vi "PECT - Scan_time gate_counter -XSeries-DAQ Pulser.vi"() -> ()   [LabVIEW 2018]
uses:
  <vilib>/DAQmx/read.llb/DAQmx Read (Counter U32 1Chan 1Samp).vi
  <vilib>/DAQmx/write.llb/DAQmx Write (Analog Wfm 1Chan NSamp).vi
  <vilib>/DAQmx/read.llb/DAQmx Read (Analog 1D DBL 1Chan NSamp).vi
  <vilib>/DAQmx/read.llb/DAQmx Read (Analog Wfm 1Chan NSamp).vi
  <vilib>/Instr/_visa.llb/VISA Configure Serial Port (Instr).vi
  <vilib>/DAQmx/create/channels.llb/DAQmx Create Channel (AI-Voltage-Basic).vi
  <vilib>/DAQmx/create/channels.llb/DAQmx Create Channel (CI-Count Edges).vi
  <vilib>/DAQmx/miscellaneous.llb/DAQmx Fill In Error Info.vi
  <vilib>/DAQmx/configure/timing.llb/DAQmx Timing (Sample Clock).vi
  <vilib>/DAQmx/configure/trigger.llb/DAQmx Start Trigger (Digital Edge).vi
  <vilib>/DAQmx/create/channels.llb/DAQmx Create Channel (AO-Voltage-Basic).vi
  Global_data.vi
  <vilib>/express/express analysis/Spectral/Block/exnSpectralBlock spectral measurements PSD poly.vi
  <vilib>/express/express analysis/Spectral/Block/exnSpectralBlock spectral measurements PSD WFM.vi
  <vilib>/express/express analysis/Spectral/XNode/ExpressSpectralMeasurementsBlockNode.xnode
  <resource>/objmgr/daqmx.rc
  <vilib>/measure/NI_MABase.lvlib
  <vilib>/Platform/NI_3dgraph.lvlib
  <vilib>/DAQmx/write.llb/DAQmx Write (Analog 1D Wfm NChan NSamp).vi
panel:
  in  "Tab Control 3":enum32{"Control", "Data Processing"}(tab)
  in  "Duty cycle %":dbl=50.0 format="%#.2f"
  in  "Pulser Trigger":tag="/Dev6/PFI0"
  in  "Edge":i32(ring)=10280 items=["Rising"=10280, "Falling"=10171]
  in  "2 Plots":bool
  in  "Offset":bool
  in  "Open csv":bool
  in  "Scan":bool
  in  "Save Scan mode":bool caption="Save Process"
  in  "Gate 1":dbl
  in  "Gate 2":dbl=50.0
  in  "Stop Scan":bool
  in  "Right":bool
  in  "Left":bool
  in  "Front":bool
  in  "Back":bool
  in  "Home X":bool
  in  "Home Y":bool
  in  "Stop 3":bool
  in  "Emergency Stop":bool
  in  "Move Distance":dbl=5.0
  in  "Pulse generator":T1={"Waveform Type"=2, "Amplitude"=10.0, "Frequency"=1000.0} {"Frequency" format="%0.2p"; "Amplitude" format="%0.2p"; "Waveform Type" items=["Sine Wave", "Triangle Wave", "Square Wave", "Sawtooth Wave"]}
  in  "Open tdms":bool
  in  "Motor Counter Terminal":tag="PFI8"
  in  "Motor counter":tag="Dev6/ctr0"
  out "Motor Pulse Count":i32
  in  "Cursor":bool=TRUE
  in  "Repair Line Col":bool
  in  "Repair Line Row":bool
  in  "Line Col":dbl=167.0
  in  "Line Row":dbl
  in  "Y-max":dbl
  in  "Y-min":dbl
  in  "X-max":dbl
  in  "X-min":dbl
  in  "Inverse":bool caption="Scan"
  in  "ViewMode":i32(ring) items=["cwViewXYPlane", "cwViewXZPlane", "cwViewYZPlane", "cwViewUserDefined"]
  in  "Plot style":i32(ring)=5 items=["cwLine"=1, "cwPoint"=2, "cwLinePoint"=3, "cwHiddenLine"=4, "cwSurface"=5, "cwSurfaceLine"=6, "cwSurfaceNormal"=7, "cwContourLine"=8, "cwSurfaceContour"=9]
  in  "ColorMapAutoScale":bool=TRUE
  in  "Max":dbl=0.6
  in  "Min":dbl=-0.8
  in  "low cutoff freq: fl":dbl=40.0 format="%0.2f"
  in  "Filter":bool caption="Scan"
  in  "Backindex":i32
  in  "Backdata":bool caption="Scan"
  in  "Odd":bool caption="Scan"
  in  "DiffX":bool caption="Scan"
  in  "DiffY":bool caption="Scan"
  in  "Abs":bool caption="Scan"
  in  "Trim data":bool caption="Scan"
  in  "Return":bool caption="Scan"
  out "Start Pos. X":dbl=-22.5 format="%#.4f"
  out "Start. Pos.Y":dbl=18.8 format="%#.4f"
  out "No.data":i32
  in  "Stop 4":bool
  in  "Tab Control 2":T2(tab)
  out "Hall sensors signal":waveform(dbl)[](graph)=[{"t0"=timestamp(3525645621.636764 s since 1904-01-01), "dt"=1.9999999999999944e-06, "Y"=array[2100 elements], "attributes"=variant("NI_ChannelName"=variant(string "Dev1/ai0"), "NI_UnitDescription"=variant(string "Volts"))}, {"t0"=timestamp(3525645621.636764 s since 1904-01-01), "dt"=1.9999999999999944e-06, "Y"=array[2100 elements], "attributes"=variant("NI_ChannelName"=variant(string "Dev1/ai0"), "NI_UnitDescription"=variant(string "Volts"))}]
  out "Feature Extraction":dbl(graph)=0.021153968958947764
  out "Power spectral density":cluster{"f0":dbl, "df":dbl, "magnitude":dbl[]}[](graph)=[{"f0"=0.0, "df"=238.09523809523876, "magnitude"=[-25.4340272409559, -28.495970805276507, -69.09064054555873, -79.11355871279994, -75.69366097931027, -84.18131507822396, -80.50168881348966, -82.72314293089615, -87.19630499623688, -82.83568021481967, -89.95290866002237, -85.90392585035596, -87.41269111550386, -91.40893948681482, -86.69370819914215, -93.36336146616782, -89.019380476413, -89.73232030153878, -94.58261196624535, -89.16287927388944, -94.965890302584, -91.86846413178648, -91.95327957161693, -97.62687167891286, -91.59993648735762, -97.30685711015555, -93.8350762480425, -93.27921214218685, -99.59438563802183, -93.1824258709588, -98.3113125531512, -95.45425138584356, -94.39327135467576, -100.65352961491782, -94.55889081970952, -99.40788907105079, -97.93617495318924, -96.19517579047603, -103.97036797797732, -96.40295202889732, -99.7036956909043, -99.48760137175819, -97.46192979187015, -106.29271483151813, -97.51447379981207, -99.86179280251669, -100.43811038443037, -97.59011642740829, -105.58363666166275, -99.01126121197593, -101.01575323613292, -101.90167607549864, -98.61952569586691, -106.73670466995647, -99.29976101634999, -101.54959604687718, -105.17330050767885, -100.09392305285375, -109.78264848704497, -100.98914236173123, -101.81665207962125, -105.42358374403365, -99.82880728595141, -107.07330885402075, -101.07712607444097, -101.03780825357597, -107.32811151840846, -101.221643458408, -105.63776326231454, -101.8420593566944, -101.80081629073969, -107.47915505307212, -101.12986632760553, -106.84901404755908, -102.73715610491038, -101.51552854007832, -107.28771371003282, -101.3928633472346, -107.44515355816633, -104.89304864643535, -103.1455098860718, -110.19910428997925, -102.73063833081197, -107.57101838377707, -104.90574568581201, -103.72599931018533, -109.97178587260123, -103.24611921258705, -108.36098023558972, -106.6408311450923, -104.73569536588386, -116.21683530762306, -105.02627439976544, -107.15856030450797, -109.81191038702062, -105.53476822084077, -119.10077766590356, -105.31867536160968, -106.9718410299748, -108.34458911268797, -104.70307996109247, -114.76704583683203, -106.29948298493936, -108.55077108437321, -112.16618350190343, -105.98453547558171, -114.68576835450673, -107.50968901677987, -107.89174277914348, -111.59875709602721, -106.69368240333122, -114.93273233954758, -105.23904516482949, -106.00272331017348, -110.36103151258544, -104.93177986717492, -110.8835476773746, -106.69346348818806, -106.66103973993782, -119.11729839814336, -108.06338160849775, -114.5879267769655, -108.59816838472844, -107.53189260743514, -114.07390818184973, -106.70996756049796, -113.27381274118753, -109.50270539577696, -107.37282420343303, -113.4779718725949, -106.04267666963091, -111.30294425571472, -112.46717993668915, -109.13164915488709, -116.65287200885172, -107.03002573045511, -110.21479040603631, -112.476075561056, -106.97710947409149, -119.42145279296255, -108.3200486628316, -110.46641858585929, -117.16650627564961, -109.73297826697552, -120.31689830731365, -107.19513745371916, -110.66663569403087, -113.30365980039964, -110.01971553524372, -123.68660617105166, -110.8171755739396, -111.11382172813546, -117.76239209582961, -109.49899370205401, -115.22252846498625, -111.1932077339224, -112.38235939086871, -118.22207022901702, -110.6546796895719, -116.97450780644367, -110.82401674194465, -111.96705198878843, -118.28092956599232, -110.5621503678909, -121.25720613496851, -111.98371482341479, -113.27928013246557, -111.96833712758355, -108.56859286664552, -120.32790468431601, -110.82699792221703, -110.79062667340345, -122.65756767769517, -110.48843456045427, -116.8782055296399, -115.43719816168479, -114.47619780315773, -121.42183196132746, -111.60631415727042, -120.68077308056417, -109.35478690141552, -109.03210709352732, -120.6260555904793, -109.47936424950136, -113.33719701518146, -112.88325992990137, -110.99901978536154, -123.19636626521421, -109.09861317900774, -113.33125158106256, -115.35673297389727, -112.77249677632989, -124.61163141716472, -114.68140920359865, -121.89642913325117, -115.47413298424323, -112.82196063671608, -127.87542521315149, -111.54178118788309, -113.6448752704395, -120.76569423868874, -112.98651214877823, -123.18868565400437, -115.41399838634062, -115.46853076016815, -116.40989072804102, -110.69611347288615, -132.23164080331392, -114.76376391429793, -121.7246597336247, -117.46893009589195, -114.01899156779395, -125.22079066032327, -114.59524199183258, -114.50034890537415, -122.9532092227648, -113.72727798159212, -125.65163915514907, -113.4793801211504, -110.4090756414644, -125.63592649005872, -114.22938378193007, -116.74947251106808, -121.60535557984142, -116.79385283402802, -122.44667696630361, -113.43873413563811, -123.28159708694415, -113.92892974938164, -114.01193823589753, -121.62751955742443, -118.76839573694522, -125.52998605097204, -115.19609643487229, -117.49409595176479, -117.08423885198002, -119.48314867245172, -125.01675515413412, -117.92668164142911, -115.55962389856793, -125.63488616674975, -119.11862859365166, -114.78860770332909, -117.18339781294443, -111.18063004722558, -118.31775966044624, -111.6867367949252, -114.57226159377, -119.36541212960576, -113.90245139442648, -132.46343443313128, -120.1282759002165, -121.05279009698619, -118.9115822659523, -121.23280439248342, -116.31914159559688, -127.38829313950257, -117.34673005740623, -115.95249861902771, -114.9301657394146, -123.22361802797445, -110.83274939062106, -116.16624248562111, -116.76753364192771, -113.94454545069023, -122.95736945775944, -118.66755800656253, -129.1462641201204, -116.6351050110328, -117.22529407303742, -123.80212197360244, -115.89792176423389, -114.25823938606595, -125.60467961977515, -114.59958849364433, -121.70071005514421, -118.25968972451209, -114.69929400946009, -123.88209034116528, -115.03869272537257, -117.52034211782204, -115.27990843516797, -117.85366603932033, -125.16865559622727, -118.21960424638507, -119.69008755413566, -117.24640963460672, -114.32867295013791, -119.1576982419508, -122.85495988425586, -116.3373010103401, -114.53730203699834, -115.67017599990201, -127.144321037601, -115.73849102686786, -117.7626163106355, -119.7346592991025, -117.41317517684553, -125.0417974461613, -114.5488949833583, -116.59812516173781, -119.91064563147799, -115.27933218667663, -122.09990513751134, -120.95678574143693, -123.25641714743752, -112.5173710452192, -113.53735878806998, -129.23914933506734, -116.27157269711533, -148.4020512032711, -118.84888216023774, -123.82550527215588, -116.87770979616658, -111.32191810025745, -124.32675905891588, -114.37182733794062, -121.10713785851372, -122.59698730059695, -116.38346694563282, -121.69144349152856, -119.00883142493832, -110.81886738196273, -120.7909830607913, -115.01780448665316, -114.52055121633796, -132.6824191654361, -116.330695115645, -126.4664151018508, -118.32717907779282, -118.7288071595281, -120.42749846140066, -112.53185615773879, -124.26026008984286, -114.24089252048742, -120.00368190003405, -114.71738500842926, -112.92262025927133, -129.21127897188563, -113.5947811765517, -117.80802009651353, -117.0133790103226, -112.19210322760304, -118.17549968071762, -119.3256187825503, -118.84981507334446, -121.39118969751144, -114.64543555194373, -119.84814933224528, -114.09123407848944, -116.22899352170892, -116.41650104077173, -113.70057202673476, -124.52773908304957, -114.87372641784933, -116.11651108221098, -121.68680962246994, -115.78306007961302, -122.22621008657796, -118.81157995182392, -113.9402115821658, -132.636729517989, -114.49554876936634, -119.50980190398928, -123.27410972236837, -118.52851881066383, -122.25212982572599, -117.13947036230024, -120.85005588797962, -118.41526503460501, -117.61788553858068, -126.3872056783977, -114.98198608543298, -119.7789938911847, -120.84873579392627, -114.38831474301695, -153.35954756825245, -113.19505610638078, -114.17454820985151, -127.41069917723112, -114.92677241657191, -125.49053973810628, -113.36382196587914, -119.96785250843519, -122.47388530423243, -116.38671253508838, -120.0905790211523, -119.83326265062107, -117.88168146696918, -122.3132169880757, -115.87324909105399, -125.92003267803432, -113.96860176867415, -114.49156118371398, -127.52634390035722, -115.05967156528004, -126.82020221981517, -117.93643187259194, -116.51163213641807, -119.47551219110167, -119.55225172256931, -116.9512257852571, -122.23153124485954, -120.8368476753637, -121.48473913072222, -115.83122660909913, -135.74260014140523, -116.58358375805423, -118.15236945484727, -119.06674062398864, -115.7844834762477, -125.06111738611818, -114.7801535050972, -115.2696605691888, -123.98656374010793, -119.29025555731172, -118.29146803784099, -119.55696172158135, -118.06884171238352, -127.81587648134607, -120.41730580797976, -123.49626136731604, -112.2147141798107, -116.22555232584983, -132.79419178871254, -119.66964883124663, -117.20946469243259, -118.20939292735417, -115.6951914646649, -129.64892855822356, -114.27056999288617, -120.31005512957381, -117.41846777372632, -115.50158386260813, -124.69777160737624, -115.2892897247205, -123.61522771666871, -113.75248734362687, -113.22999749252833, -129.3490509395313, -116.88137735661701, -116.94110280242681, -119.50244079984806, -119.30521139999144, -128.17199984115797, -118.06736594940236, -116.05331575995922, -121.29670750650897, -116.1140297602044, -125.090619084802, -121.41807296062154, -120.01332757902264, -120.54914530643151, -116.49738633175463, -122.32551291835904, -118.3190808346865, -118.92638453656723, -122.48819531011718, -117.01021725424317, -120.98896352560598, -117.23831688685218, -121.27915259197124, -121.20017251921661, -117.6155648860373, -120.91300272912063, -117.94438460863424, -115.94437430101533, -123.35904829443987, -117.74011174503076, -121.54935745388448, -120.82564553545025, -121.98951430455743, -120.24858103448778, -116.44403527138395, -112.79571494351876, -112.42801913096545, -110.1697573019791, -115.34500457736401, -119.81921052956707, -129.82600951154313, -115.5862301263047, -112.59292882433087, -120.79009137478283, -131.32849293387295, -113.61194478398238, -123.48568856527031, -119.17507777781304, -123.09261867490484, -116.97755217417308, -123.94453461434183, -116.58080525616379, -119.64289646280756, -122.90202645580743, -126.66219093058154, -121.95048829056148, -115.72578023509817, -116.70117814464484, -121.91050280869723, -118.25299095698178, -116.45905559047064, -132.57794493731578, -121.65327820443292, -120.9816664775787, -117.17270262269045, -120.27433984830965, -125.89418976028173, -119.09563505847817, -126.9693215534833, -113.17465524665704, -118.98702092883116, -119.83822568580342, -120.45832738089722, -120.67735960513633, -127.38676010839353, -127.65777338183055, -118.37446329057411, -115.61355494839711, -119.94568688114103, -116.06619937633681, -126.348857777089, -118.92850079147068, -119.5416617639739, -132.47075644221843, -118.08809356028496, -123.16186463092723, -121.51579486791232, -122.88983670053283, -129.5195538417256, -120.4730389608841, -132.16486858341602, -122.34690358436781, -120.71922104337597, -114.29260860841114, -117.67902631803368, -124.7040155514909, -123.51274592117205, -120.02297921674332, -136.54655493811157, -120.45629227407751, -119.06410204276258, -127.91681714792554, -122.82090055753153, -125.16838176650813, -121.79565386970478, -119.79607311590995, -126.54861375039647, -121.59135878113302, -132.8348640697562, -118.1305434733294, -120.46070148841905, -122.69571910896963, -117.6534954653865, -124.15742546824006, -120.73646926947502, -124.82696993800742, -124.513836786494, -123.15395713389651, -124.62395468806395, -117.21365768658171, -119.32635871968456, -121.48532284413152, -119.38242892643675, -126.25575652510352, -123.27133124029851, -117.58533922728374, -118.17710108929799, -114.99496360200965, -117.77133194647278, -111.34898201101595, -111.50817058307922, -119.0703124690998, -127.70676079885351, -121.8704969141074, -125.93154214283446, -118.65628450081473, -122.47918878348962, -117.9651589546518, -126.13560583004508, -122.42294805637847, -133.924453763793, -117.2082573038767, -117.6525335446734, -122.92077297426977, -122.04624645756786, -116.43289028226238, -117.93180959338378, -129.02356734231915, -117.95493621286326, -120.7555929766252, -120.76782849311112, -123.06287498470708, -117.83798593857965, -123.43423215434719, -120.15190119516652, -120.48240443128407, -143.29738987393452, -123.46572247444769, -120.89055325172792, -125.66715973809033, -118.26887578998644, -117.01836200028421, -121.33021830755509, -119.68846363313813, -122.60689066103069, -116.26858138914181, -119.59360791972998, -122.94866175463353, -114.174409515556, -118.00516930888391, -121.56978543579633, -135.87799017759036, -117.50816594504829, -122.82539428457626, -123.82103443155845, -124.77975840345442, -121.13340798086698, -120.93607435603558, -133.15787160745222, -120.70545628137863, -125.02155972441679, -122.04666465472178, -118.01234649746348, -127.88767491042842, -119.02096620167217, -120.16031065152875, -122.25406107859625, -121.72733059051095, -120.61357375519918, -118.63962847172827, -134.3857741605498, -116.3600853185034, -117.26695700691671, -119.9176982185873, -113.45576465218444, -126.69779573632724, -114.39554522802246, -116.8457146515868, -116.34219889483086, -119.30011291548334, -120.01163291843496, -114.29497178248809, -127.65687642749229, -119.58556923753022, -129.8593054181261, -122.2353645100479, -120.79536520223796, -119.83284028355028, -117.7991246185715, -128.390292904734, -119.78079925213122, -125.478913448993, -113.89747777944768, -112.66620124153357, -124.3475049842711, -120.85847303094337, -132.91807981902295, -119.523494985723, -116.65149909866443, -119.73287290436721, -127.63237851524192, -127.23413304048789, -120.87585453904362, -121.08540368080186, -134.91071939669257, -117.75375801669338, -117.2683014590723, -120.9739099492833, -118.23809733632451, -120.94065804928206, -123.88077510875804, -118.13812819300607, -122.60294123365466, -126.97075898006995, -120.18754789731035, -124.71238663441227, -120.55456557278582, -130.94599087480253, -111.18288669417035, -112.27708791831247, -126.0512034600378, -117.41881712783596, -128.20553880273903, -117.29482600885808, -118.2045526390752, -127.81966672699878, -117.03716165902529, -115.46711739757512, -117.15363929234843, -121.87599671671335, -121.19736800869221, -126.5301786755875, -131.20754947382918, -124.40138004810741, -129.0562496906515, -121.06816554587536, -121.01023627802867, -138.6137911215848, -120.12495002524031, -121.38510517514229, -122.79804220535513, -116.97501378195477, -118.82011581137473, -114.0229185604644, -119.54287501990726, -114.64474566771625, -117.76935669872461, -123.81082574158907, -118.51678358865587, -128.9664755188374, -123.45357998434133, -122.74888841574231, -120.74640581234044, -126.956344345126, -119.95682140104577, -118.8873101779055, -124.41062359284174, -128.97304498664363, -123.86287113204068, -127.30257087528216, -120.61364220528216, -114.45119129304715, -119.68384044686806, -131.29639185291157, -122.31250766293485, -119.57420865241102, -124.74014026002448, -124.87593035709094, -118.4566565612952, -123.76236085976001, -120.84780538841838, -117.68987599773281, -135.06195695255914, -122.56143585795171, -129.04610316842883, -118.32313199570537, -117.77093802786419, -124.46572845786741, -129.1123298336903, -120.88470269965448, -116.69988985752187, -116.84054667499878, -133.76883696987278, -122.32434984927302, -124.98940594457933, -122.56515592789917, -118.31562562243366, -133.97049179545627, -122.33220627999802, -131.16753675316977, -124.69828063969263, -116.37621154460467, -126.1833423168025, -129.62937634161355, -118.46241371150788, -117.52851478852457, -125.32425037236442, -119.0327364293772, -124.2861355894013, -123.24573502278234, -125.52155812053758, -113.75743410709823, -114.79513162658353, -128.58142362588052, -122.48277095196701, -118.94747544412269, -123.86988127835491, -124.78140456983323, -121.53998481875398, -116.01432822539552, -119.20174681160661, -122.75167725800814, -120.58657749420254, -118.51141061842183, -119.24457006171983, -131.43641234223372, -116.00759139055087, -121.24442216102587, -123.29371279953725, -117.608355420454, -116.33684374617326, -118.06291688281922, -121.88761866022774, -121.54820313120047, -119.5051369873635, -126.56611158390913, -118.84012713615805, -121.09285296522563, -124.67955377692547, -147.31451139022337, -116.80660421066897, -114.8367853755961, -120.41026468628925, -123.65666101895222, -119.64837119787269, -116.77480172559095, -116.54263359173909, -124.75286620868079, -117.33721912698883, -116.51795620907136, -118.50086748176733, -128.10381328920522, -122.78098994574157, -120.24716756092855, -119.52743204722819, -115.00407387659232, -108.2853711552629, -108.61086943894702, -119.6228894146785, -124.11132022420912, -125.6202218409766, -123.1749360787656, -118.1971196161698, -123.95075368058998, -121.72140109898365, -123.27106899042522, -123.73035629887062, -121.24369679109273, -121.07381526465288, -113.13965659723667, -118.330755475899, -118.40249076804484, -111.59630598649044, -116.1569506845575, -125.67326089915758, -125.85723567111906, -119.24293277595024, -117.87067617433537, -120.70936924059559, -131.8090588468898, -132.98711569625004, -123.63274249467587, -122.75476917502559, -126.12873814250243, -120.53144270605179, -129.07030822919336, -122.7889410422919, -124.35405971166259, -119.63968579420454, -139.0154441054289, -129.47962001806934, -121.86548015410847, -128.6818469257012, -121.40195873232601, -138.64231053781285, -124.22025721762265, -124.06073958736941, -126.71929802352521, -131.7498459276443, -120.68144109742178, -122.6325588818875, -126.80796617875095, -124.92487955227033, -136.94498040498806, -124.26704334219014, -123.21376211221711, -140.25352033075964, -129.53222319772195, -122.58541579060463, -122.1996729592375, -125.66642108013673, -125.66310429236694, -120.09682773706965, -125.27326633941439, -121.55721878725502, -121.22507119941083, -121.53716878624485, -136.20685498111987, -128.15260146013156, -120.03473972471616, -124.60755958763912, -124.73082500077143, -123.93425949983688, -131.04483249265184, -121.7957035014449, -127.09321441816094, -133.6144579272493, -124.69014595896968, -130.4902091211609, -121.18031440773905, -128.00033943961677, -125.88991118115149, -118.865310745079, -123.69668867733147, -117.98756965862728, -114.40013091842827, -118.28685032521078, -122.23464196869948, -124.8440422629961, -129.66281606870848, -119.440534215621, -124.54391783563877, -124.93447967158188, -121.7258558761523, -122.28817885403082, -127.06889620458577, -128.92172974939206, -120.62932166634072, -126.06847321900452, -123.31471168429935, -121.80350826545656, -129.2574604322076, -125.67225933193998, -125.7801671825605, -129.53804733161627, -119.56756644124712, -128.82490314699373, -124.7689736295626, -120.50019729114693, -124.50603158563972, -122.8120627011088, -125.60528875555717, -123.8817354922713, -124.05570537836674, -120.94568834491936, -118.06056028605255, -124.24390361274648, -125.5716703018188, -127.71949519914061, -130.7001652968252, -126.27701412017494, -133.76810134709916, -128.4738939614179, -120.302550881701, -118.91298143662928, -124.9077318110765, -127.16253699189492, -118.11405934812818, -117.52028071290711, -140.95620572748925, -123.61977932545628, -131.0334379970501, -125.88948384968432, -127.81552331993379, -121.92316280719056, -119.05911238768732, -126.83773251459189, -123.52627415002164, -120.8779561023192, -123.66683567603742, -131.64300993967345, -123.62895847772963, -116.89792951363142, -120.1068259250195, -117.92484706459337, -115.58208487778379, -120.76803581628594, -123.95408562090736, -122.79456549632754, -134.5305398779298, -123.57040300991032, -128.40634159414552, -123.70102187824159, -118.24970739397313, -119.66483900349026, -127.78024313111393, -120.3547204111785, -125.49305364308705, -119.49505591004302, -120.50920386196539, -119.03509516851003, -114.24667300009652, -121.60538636584391, -119.95304417598024, -122.24585853682832, -128.63653016912684, -116.04810628805795, -121.94159862131235, -122.59928204398939, -121.4532410501923, -128.6511474663462, -130.83715595958148, -121.71998300574741, -116.91426629511156, -113.587592058512, -115.59736707638731, -124.65300822631244, -133.32538684258748, -124.02289142873636, -121.54278890993639, -119.02596809402394, -108.90572887117857, -112.14974069608851, -129.21149299565423, -118.82148342951197, -116.65510894288538, -118.39609618084175, -116.53502642884725, -122.47549439965209, -122.23125657046063, -123.68081343116663, -120.67915071600007, -123.6899360128769, -118.56721985209728, -118.36641581191942, -126.96724630704657, -119.36877661672403, -123.07698921198843, -117.80772421906035, -122.82545076270567, -118.82755071380888, -117.21030132539394, -129.760567864525, -118.0816708063509, -125.80573274113647, -121.18434666182338, -121.80987210832065, -130.99259828357094, -125.47223579895922, -123.86818606677002, -118.7118158196511, -119.27778317338742, -127.27333258839096, -119.90672352079164, -140.78772370844268, -118.08251080057329, -119.86636232122572, -118.69482489738232, -119.19106512767372, -123.70988914879189, -121.92566832147995, -123.41378261726373, -120.1715186070818, -117.9079629421116, -117.41960207545632, -123.72833996166874, -127.24377206607298, -124.99098647980887, -129.48803701799955, -129.92351350561592, -120.79284154834647, -119.29601975194524, -136.17244775530037, -126.73975437546255, -128.84068276143336, -125.66374985701982, -136.69026010435715, -125.44409235146617, -119.28138070315057, -118.65017329869724, -118.02521532826772, -122.23736063759657, -121.27846943548622, -116.69850478126861, -119.7711336696722, -123.70776561180185, -118.43344549561263, -123.92390877157247, -117.19637143066551, -117.64112988205311, -127.78399195238529]}, ...(2 in all)]
  in  "3D Surface":refnum<k7>(container)
  out "Record path":path caption="selected path"
  out "Feature extraction scan":dbl[](graph)
  in  "Tab Control":T3(tab)
  out "Completed":bool
  in  "Step X":dbl=0.1
  out "Move X":bool
  in  "Direction (+)":bool=TRUE
  in  "Step Y":dbl=0.1
  in  "Y-length":dbl=10.0
  in  "X-length":dbl=5.0
  in  "Save Speed":bool
  in  "Cur. Pos Y":dbl=18.8 format="%#.4f"
  in  "Cur. Pos X":dbl=-22.5 format="%#.4f"
  in  "Travel per Pulse (mm)":dbl=0.002
  in  "2 Rate":dbl=0.2
  in  "1 Rate":dbl=0.2
  in  "2 Min":dbl=1.0
  in  "1  Max":dbl=8.0
  in  "2 Max":dbl=8.0
  in  "1 Min":dbl=1.0
  in  "Parity":u16(ring) items=["None", "Odd", "Even", "Mark", "Space"]
  in  "stop bits":u16(ring)=10 items=["1.0"=10, "1.5"=15, "2.0"=20]
  in  "Data bits":u16=8 min=5 max=8 step=1
  in  "Baud Rate":u32=9600
  in  "COM Port":refnum<visa-resource-name>="COM3"
  out "No. X":i32
  out "No. Y":i32
  in  "DAQ Pulser":bool
  out "Sample per Channel AI":dbl
  out "Sample per Channel AO":dbl
  in  "Pulser Cycles":i32=10
  out "Actual Sample Rate":dbl=500000.0 format="%0.2f"
  in  "Physical Channel":tag="Dev6/ai0"
  in  "Min Voltage":dbl=-10.0
  in  "Max Voltage":dbl=10.0
  in  "Terminal Configuration":i32(ring)=10083 items=["default"=-1, "RSE"=10083, "NRSE"=10078, "Differential"=10106, "Pseudodifferential"=12529]
  in  "Sample Clock Source 2":tag="OnboardClock"
  in  "Sample Rate":dbl=450000.0
  out "Actual Sample Rate 2":dbl=800000.0 format="%0.2f"
  in  "Physical Channel(s)":tag="Dev6/ao1"
  in  "Min Voltage 2":dbl=-10.0
  in  "Max Voltage 2":dbl=10.0
  in  "Sample Clock Source":tag="OnboardClock"
  in  "Sample Rate 2":dbl=800000.0
  # "Pulse Shape"
  # "Trigger Settings"
  # "Data Processing"
  # "Time gate = %T/2"
  # "3D Surface"
  # "Process"
  # "Repair line"
  # "Hall Sensors Signal"
  # "Feature Extraction"
  # "Power Spectal Density"
  # "COM Setting"
  # "Speed Setting"
  # "Scan Setting"
  # "Pulser Channel"
  # "Pulser Timming"
  # "Sensor Channel"
  # "DAQ Timming"
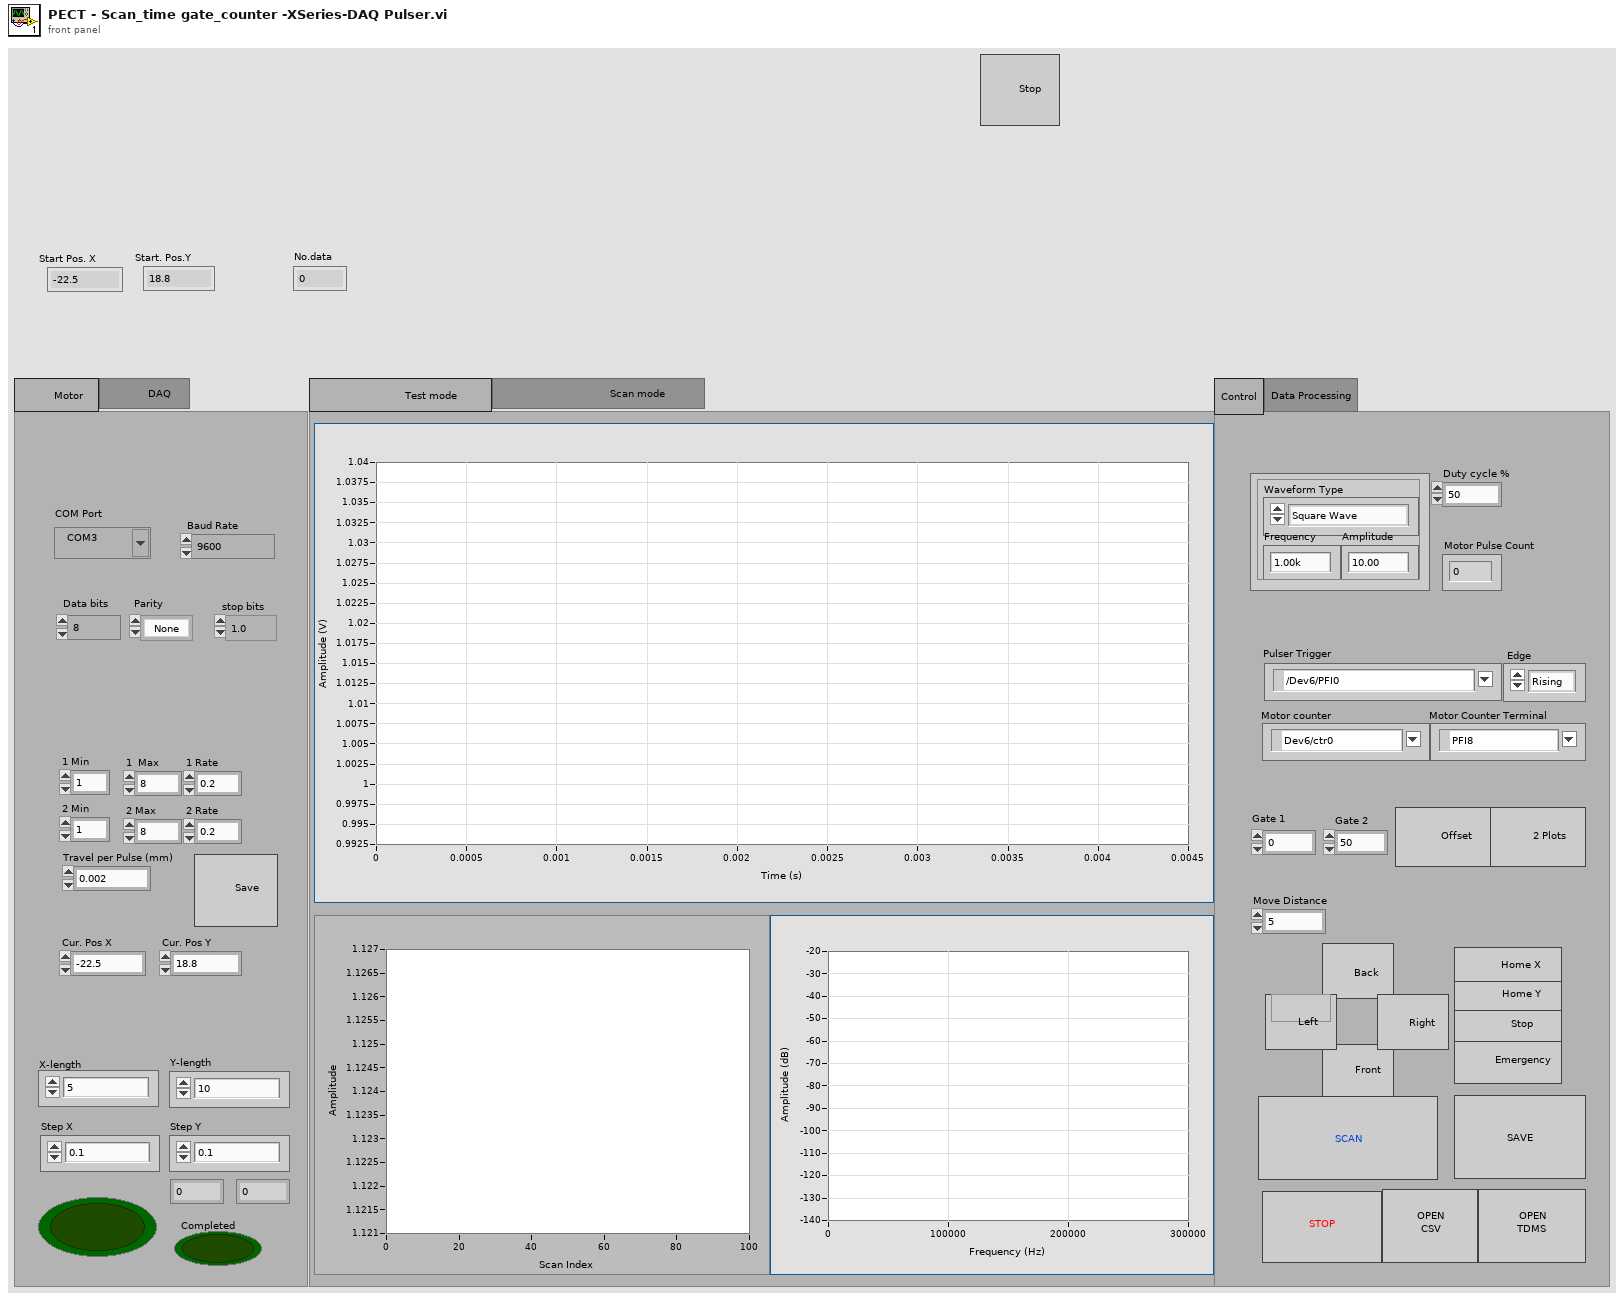
[diagram p1: front panel]
types:
  T1 = cluster{"Waveform Type":u16, "Amplitude":dbl, "Frequency":dbl}
  T2 = enum32{"                    Test mode                   ", "                          Scan mode                      "}
  T3 = enum32{"        Motor      ", "          DAQ        "}
  T4 = enum16{"No Scan", "Move X", "Wait to destination X", "Move Y", "Wait to destinatioin Y"}
  T5 = enum16{"open", "open or create", "create or replace", "create", "open (read-only)"}
  T6 = cluster{"averaging mode":u16, "weighting mode":u16, "number of averages":u32}
  T7 = cluster{"dB On (F)":bool, "unwrap phase (F)":bool, "convert to degree (F)":bool}
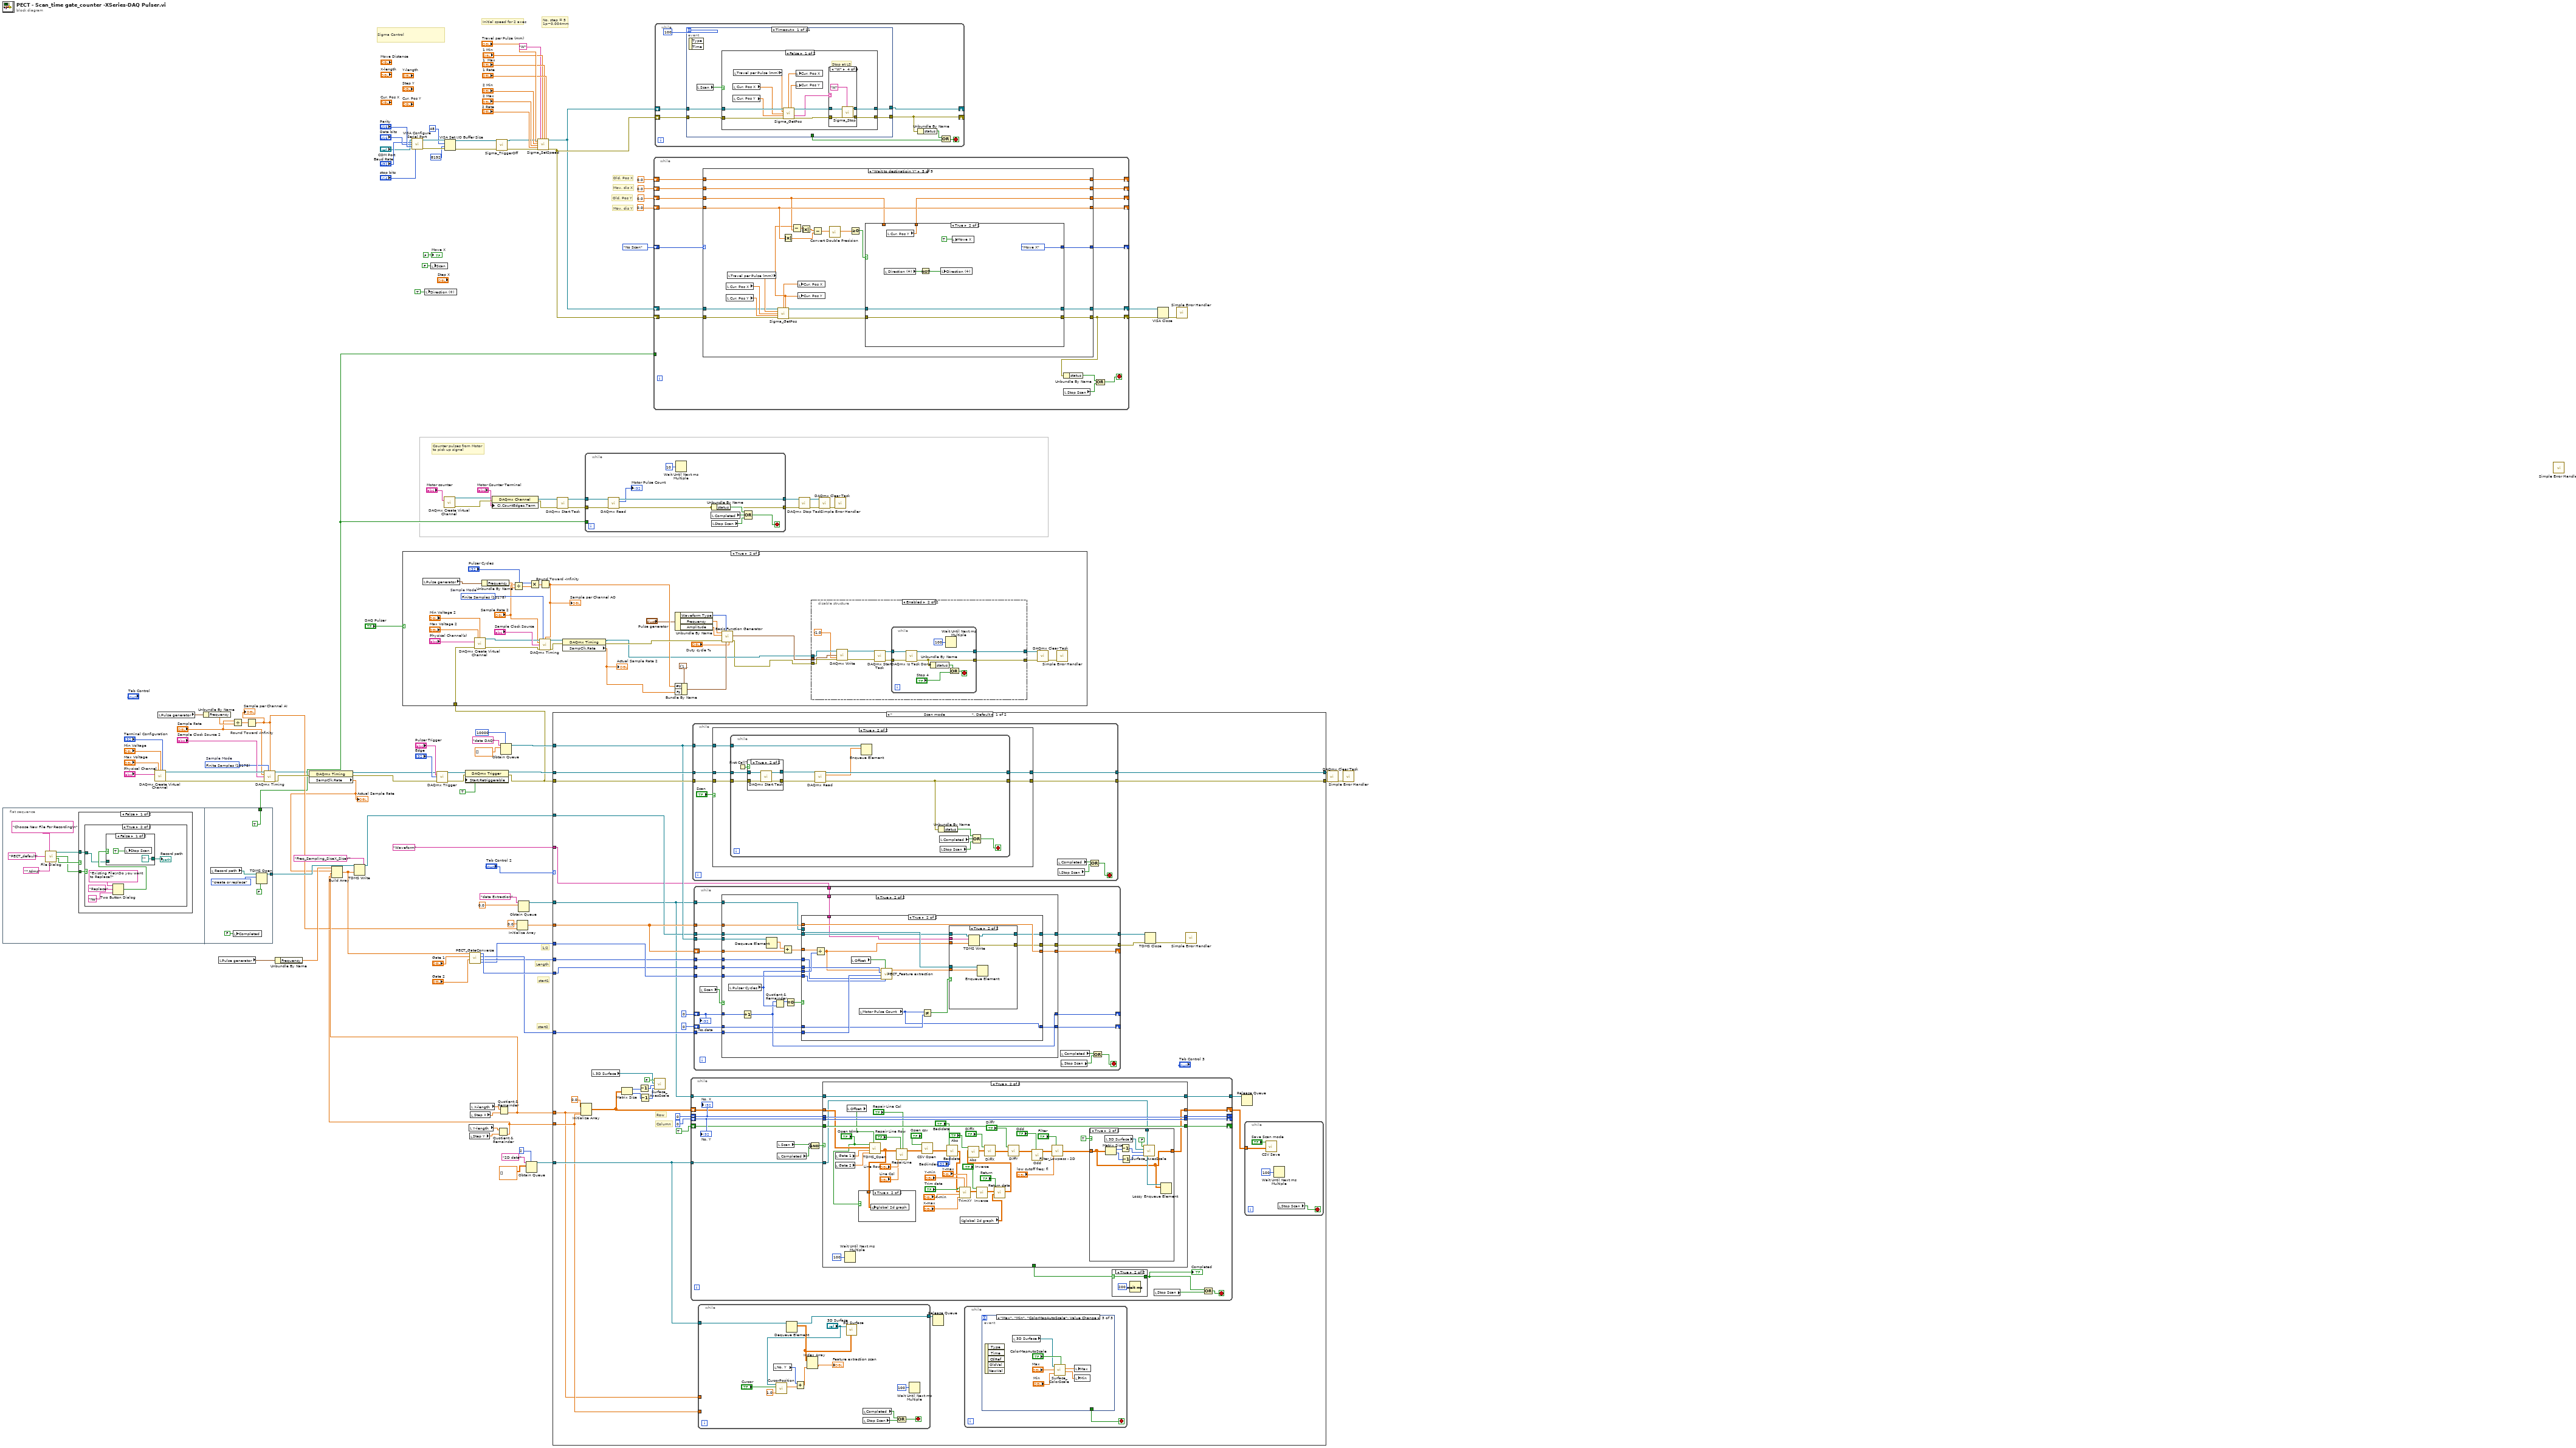
[diagram p0: block diagram]
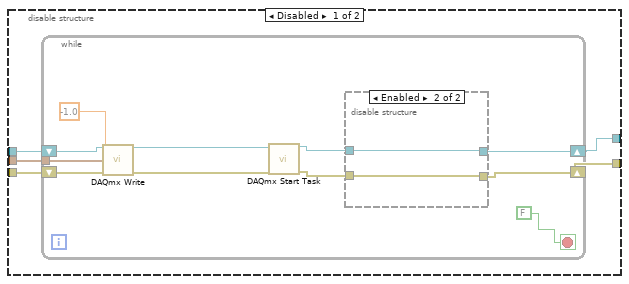
[diagram p3: hidden frame]
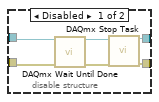
[diagram p4: hidden frame]
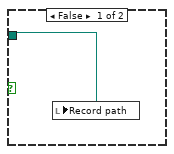
[diagram p5: hidden frame]
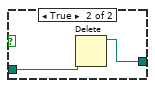
[diagram p6: hidden frame]
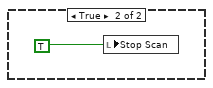
[diagram p7: hidden frame]
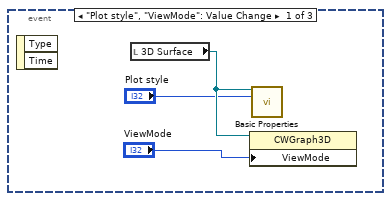
[diagram p8: hidden frame]
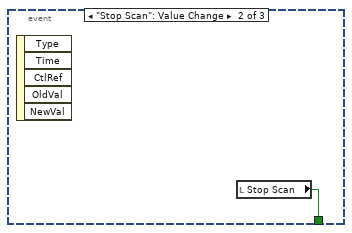
[diagram p9: hidden frame]
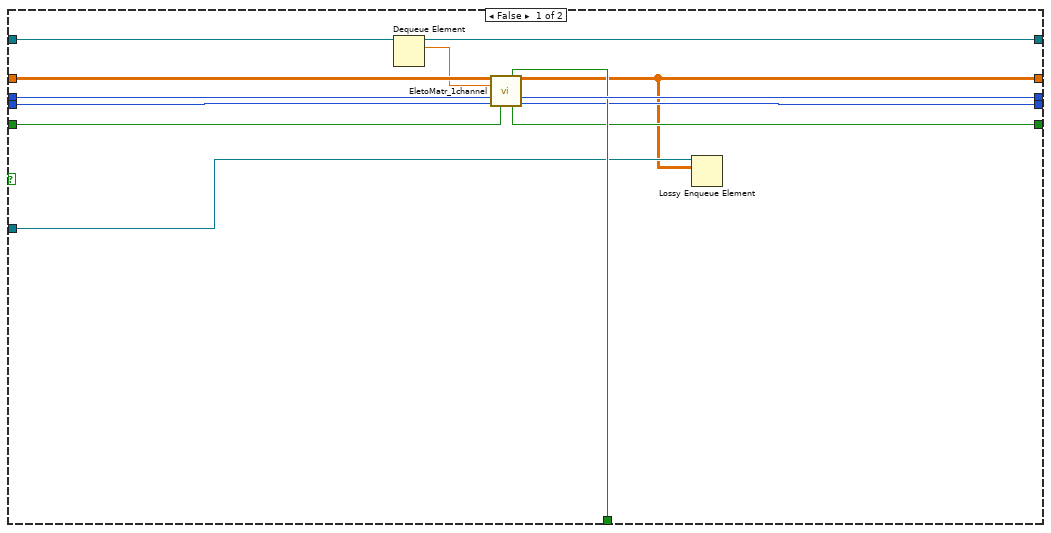
[diagram p11: hidden frame]
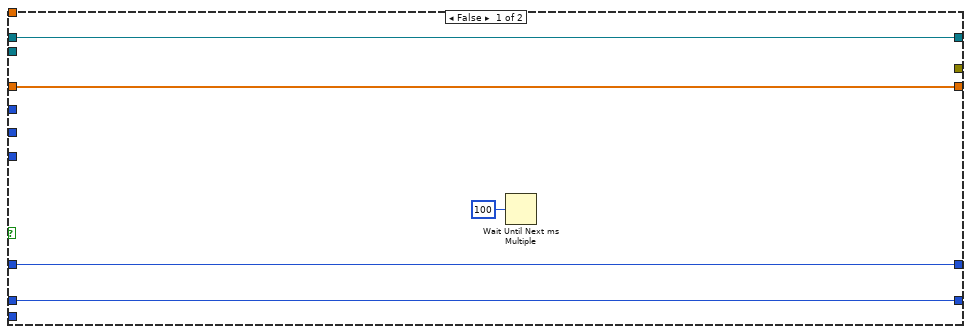
[diagram p16: hidden frame]
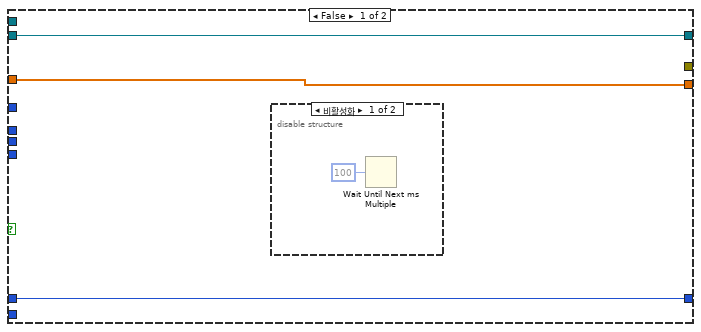
[diagram p17: hidden frame]
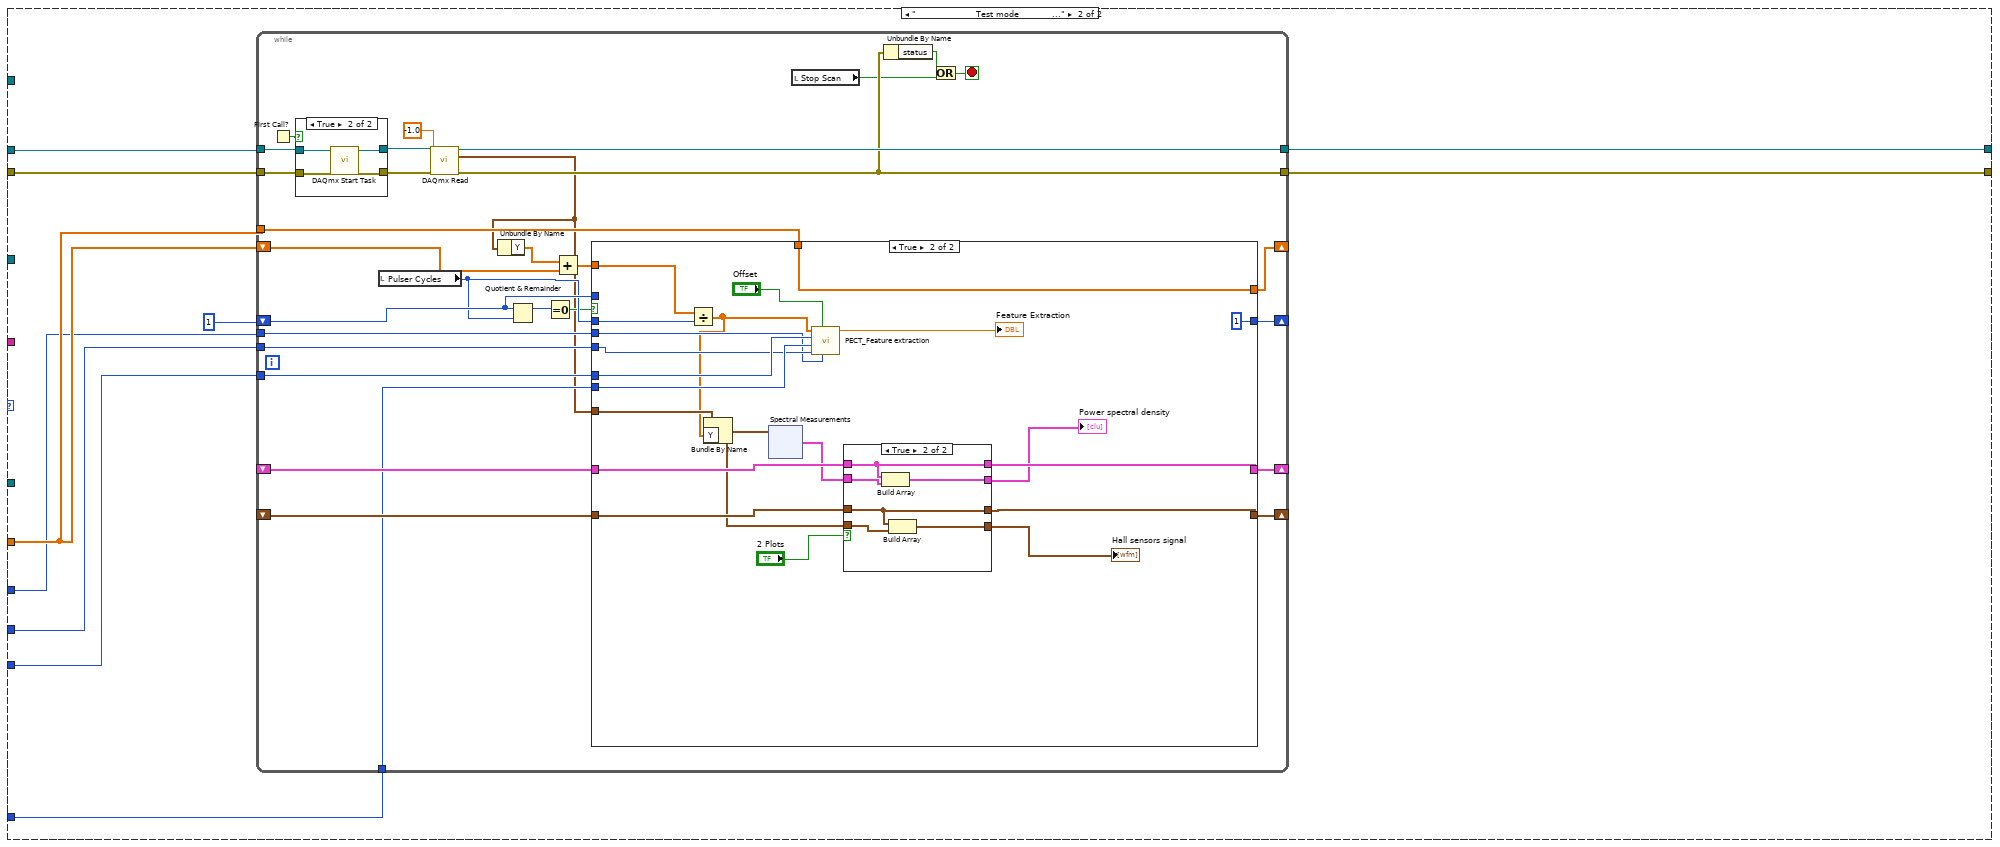
[diagram p20: hidden frame]
diagram:
  w72 = 10178 items=["Finite Samples"=10178, "Continuous Samples"=10123, "Hardware Timed Single Point"=12522]  # Sample Mode
  # "Counter pulses from Motor\nto pick up signal"
  # "1/2"
  # "start1"
  # "start2"
  # "Length"
  # "Mov. dis Y"
  # "Old. Pos Y"
  # "Mov. dis X"
  # "Old. Pos X"
  # "No. step = 5\n1p~0.004mm"
  # "Initial speed for 2 axes"
  # "Sigma Control"
  n1 = flat-sequence {
    tunnel: [w134] -> w49
    tunnel: [TRUE ("disable buffering (T)")] -> w6
    frame #0 {
      n2 = call "File Dialog"("prompt"="Choose New File For Recording\n" ("button label"), "default name"="PECT_default", "pattern (all files)"="*.tdms") -> ("selected path"=w116:path, "exists"=w111:bool, "cancelled"=w112:bool)  [unwired: 9 in, 1 out]
      n3 = case shown="False" w112 {
        tunnel: w116 -> [w117 _]
        tunnel: w111 -> [w118 _]
        frame False {
          n4 = case shown="True" w118 {
            tunnel: w117 -> [w119 w120]
            frame False {
              n5 = local write "Record path"(w119) -> ()
            }
            frame True {
              n6 = Two Button Dialog(message="Existing File\nDo you want to Replace?", 1:"No" ("F button name (\"Cancel\")"), 2:"Replace" ("T button name (\"OK\")")) -> (T button?=w121:bool)
              n7 = case shown="False" w121 {
                tunnel: w120 -> [_ w129]
                tunnel: [path "" ("deleted path") w128] -> w122
                frame False {
                  n8 = local write "Stop Scan"(TRUE ("Exit")) -> ()
                }
                frame True {
                  n9 = Delete(path (use dialog)=w129) -> (deleted path=w128:path)  [unwired: 4 in, 2 out]
                }
              }
              "Record path" <- w122
            }
          }
        }
        frame True {
          n10 = local write "Stop Scan"(TRUE ("Exit")) -> ()
        }
      }
    }
    frame #1 {
      n11 = local read "Record path"() -> (w133:path)
      n12 = local write "Completed"(FALSE ("Completed")) -> ()
      n13 = TDMS Open(6:FALSE ("disable buffering (T)"), 10:T5."create or replace" ("operation"), 11:w133) -> (3:w134:refnum<k34>)  [unwired: 4 in, 1 out]
    }
  }
  n14 = call-poly <vilib>:"DAQmx Create Virtual Channel.vi"("maximum value"="Max Voltage", "minimum value"="Min Voltage", "input terminal configuration"="Terminal Configuration", "physical channels"="Physical Channel") -> ("task out"=w82:refnum<k21>, "error out"=w83:errorcluster)  [unwired: 10 in]
  n15 = local read "Pulse generator"() -> (w33:T1)
  n16 = Unbundle By Name(w33) -> ("Frequency"=w53:dbl)
  n17 = local read "Pulse generator"() -> (w32:T1)
  n18 = Divide(x="Sample Rate", y=w53) -> (x/y=w52:dbl)
  n19 = Round Toward -Infinity(1:w52) -> (0:w44:dbl)
  "Sample per Channel AI" <- w44
  n20 = call-poly <vilib>:"DAQmx Timing.vi"("task/channels in"=w82, "sample mode"=w72, "samples per channel"=w44, "rate"="Sample Rate", "source"="Sample Clock Source 2", "error in"=w83) -> ("task out"=w4:refnum<k21>, "error out"=w84:errorcluster)  [unwired: 8 in]
  n21 = Unbundle By Name(w32) -> ("Frequency"=w45:dbl)
  n22 = property class="DAQmx Timing"(reference=w4, error in=w84) -> (reference out=w2:refnum<k21>, error out=w1:errorcluster, "SampClk.Rate"=w10:dbl)
  "Actual Sample Rate" <- w10
  n23 = call-poly "VISA Configure Serial Port"("VISA resource name"="COM Port", "baud rate (9600)"="Baud Rate", "data bits (8)"="Data bits", "parity (0:none)"="Parity", "stop bits (10: 1 bit)"="stop bits") -> ("VISA resource name out"=w97:refnum<visa-resource-name>, "error out"=w103:errorcluster)  [unwired: 9 in]
  n24 = local write "Direction (+)"(TRUE ("Scan")) -> ()
  n25 = local write "Scan"(FALSE ("Scan")) -> ()
  n26 = call-poly <vilib>:"DAQmx Trigger.vi"("task/channels in"=w2, "source"="Pulser Trigger", "edge"="Edge", "error in"=w1) -> ("task out"=w69:refnum<k21>, "error out"=w68:errorcluster)  [unwired: 10 in]
  n27 = call-poly <vilib>:"DAQmx Create Virtual Channel.vi"("counter"="Motor counter") -> ("task out"=w25:refnum<k21>, "error out"=w27:errorcluster)  [unwired: 13 in]
  n28 = VISA Set I/O Buffer Size(VISA resource name=w97, mask (16)=48, size (4096)=u32 8192, error in (no error)=w103) -> (VISA resource name out=w19:refnum<visa-resource-name>, error out=w18:errorcluster)
  n29 = property class="DAQmx Trigger"(reference=w69, error in=w68, "Start.Retriggerable"=TRUE) -> (reference out=w51:refnum<k21>, error out=w9:errorcluster)
  n30 = case shown="True" "DAQ Pulser" {
    tunnel: w9 -> [_ w168]
    frame False {
    }
    frame True {
      w165 = 10178 items=["Finite Samples"=10178, "Continuous Samples"=10123, "Hardware Timed Single Point"=12522]  # Sample Mode
      n31 = local read "Pulse generator"() -> (w139:T1)
      n32 = call-poly <vilib>:"DAQmx Create Virtual Channel.vi"("maximum value"="Max Voltage 2", "minimum value"="Min Voltage 2", "physical channels"="Physical Channel(s)", "error in"=w168) -> ("task out"=w154:refnum<k21>, "error out"=w153:errorcluster)  [unwired: 10 in]
      n33 = Unbundle By Name(w139) -> ("Frequency"=w150:dbl)
      n34 = Divide(x="Sample Rate 2", y=w150) -> (x/y=w148:dbl)
      n35 = Multiply(x="Pulser Cycles", y=w148) -> (x*y=w146:dbl)
      n36 = Round Toward -Infinity(1:w146) -> (0:w145:dbl)
      "Sample per Channel AO" <- w145
      n37 = call-poly <vilib>:"DAQmx Timing.vi"("task/channels in"=w154, "sample mode"=w165, "samples per channel"=w145, "rate"="Sample Rate 2", "source"="Sample Clock Source", "error in"=w153) -> ("task out"=w167:refnum<k21>, "error out"=w166:errorcluster)  [unwired: 8 in]
      n38 = property class="DAQmx Timing"(reference=w167, error in=w166) -> (reference out=w138:refnum<k21>, error out=w159:errorcluster, "SampClk.Rate"=w157:dbl)
      "Actual Sample Rate 2" <- w157
      n39 = Unbundle By Name("Pulse generator") -> ("Waveform Type"=w144:u16, "Frequency"=w143:dbl, "Amplitude"=w141:dbl)
      n40 = Bundle By Name(cluster=cluster{"Fs":dbl, "#s":dbl} {"Fs"=1000.0, "#s"=1000.0} ("sampling info"), "#s"=w145, "Fs"=w157) -> (w156:cluster{"Fs":dbl, "#s":dbl})
      n41 = call <vilib>:"Basic Function Generator.vi"("square wave duty cycle (%)"="Duty cycle %", "sampling info"=w156, "signal type"=w144, "error in (no error)"=w159, "amplitude"=w141, "frequency"=w143) -> ("error out"=w137:errorcluster, "signal out"=w155:waveform(dbl))  [unwired: 3 in, 1 out]
      n42 = disable-structure shown="Enabled" {
        disable-tunnel: w155 -> [w173 w196]
        disable-tunnel: [w172 w195] -> w152
        disable-tunnel: [w171 w194] -> w151
        disable-tunnel: w138 -> [w170 w198]
        disable-tunnel: w137 -> [w169 w197]
        frame Disabled {
          n43 = while {
            tunnel: w173 -> [w184]
            shift-right: [w180] -> w172
            shift-left: w170 -> [w178]
            shift-right: [w179] -> w171
            shift-left: w169 -> [w177]
            stop <- FALSE stop-if-true
            n44 = call-poly <vilib>:"DAQmx Write.vi"("task/channels in"=w178, "data"=w184, "timeout"=-1.0, "error in"=w177) -> ("task out"=w183:refnum<k21>, "error out"=w182:errorcluster)  [unwired: 9 in, 1 out]
            n45 = call <vilib>:"DAQmx Start Task.vi"("task/channels in"=w183, "error in"=w182) -> ("task out"=w176:refnum<k21>, "error out"=w175:errorcluster)  [unwired: 12 in]
            n46 = disable-structure shown="Enabled" {
              disable-tunnel: [w190 w192] -> w180
              disable-tunnel: [w189 w191] -> w179
              disable-tunnel: w176 -> [w188 w192]
              disable-tunnel: w175 -> [w187 w191]
              frame Disabled {
                n47 = call <vilib>:"DAQmx Wait Until Done.vi"("task/channels in"=w188, "error in"=w187) -> ("task out"=w186:refnum<k21>, "error out"=w185:errorcluster)  [unwired: 12 in]
                n48 = call <vilib>:"DAQmx Stop Task.vi"("task/channels in"=w186, "error in"=w185) -> ("task out"=w190:refnum<k21>, "error out"=w189:errorcluster)  [unwired: 12 in]
              }
              frame Enabled {
              }
            }
          }
        }
        frame Enabled {
          n49 = call-poly <vilib>:"DAQmx Write.vi"("task/channels in"=w198, "data"=w196, "timeout"=-1.0, "error in"=w197) -> ("task out"=w200:refnum<k21>, "error out"=w202:errorcluster)  [unwired: 9 in, 1 out]
          n50 = call <vilib>:"DAQmx Start Task.vi"("task/channels in"=w200, "error in"=w202) -> ("task out"=w199:refnum<k21>, "error out"=w201:errorcluster)  [unwired: 12 in]
          n51 = while {
            tunnel: w199 -> [w210]
            tunnel: w201 -> [w209]
            tunnel: [w207] -> w194
            tunnel: [w208] -> w195
            stop <- w203 stop-if-true
            n52 = call <vilib>:"DAQmx Is Task Done.vi"("task/channels in"=w210, "error in"=w209) -> ("task out"=w208:refnum<k21>, "error out"=w207:errorcluster)  [unwired: 11 in, 1 out]
            n53 = Unbundle By Name(w207) -> ("status"=w204:bool)
            n54 = Wait Until Next ms Multiple(millisecond multiple=u32 100) -> ()  [unwired: 1 out]
            n55 = Compound Arithmetic op=OR(w204, "Stop 4") -> (w203:bool)
          }
        }
      }
      n56 = call <vilib>:"DAQmx Clear Task.vi"("task in"=w152, "error in"=w151) -> ("error out"=w164:errorcluster)  [unwired: 13 in]
      n57 = call <vilib>:"Simple Error Handler.vi"("error in (no error)"=w164) -> ()  [unwired: 4 in, 5 out]
    }
  }
  n58 = local read "Y-length"() -> (w56:dbl)
  n59 = local read "Step Y"() -> (w57:dbl)
  n60 = local read "X-length"() -> (w59:dbl)
  n61 = local read "Step X"() -> (w58:dbl)
  n62 = property class="DAQmx Channel"(reference=w25, error in=w27, "CI.CountEdges.Term"="Motor Counter Terminal") -> (reference out=w20:refnum<k21>, error out=w21:errorcluster)
  n63 = call "Sigma_TriggerOff.vi"("error in (no error)"=w18, "VISA resource name"=w19) -> ("error out"=w16:errorcluster, "VISA resource name out"=w17:refnum<visa-resource-name>)  [unwired: 8 in]
  n64 = Quotient & Remainder(x=w56, y=w57) -> (floor(x/y)=w5:dbl)  [unwired: 1 out]
  n65 = Quotient & Remainder(x=w59, y=w58) -> (floor(x/y)=w47:dbl)  [unwired: 1 out]
  n66 = Build Array(w45, w10, w47, w5) -> (w15:dbl[])
  n67 = TDMS Write(0:w49, 5:"Freq_Sampling_SizeX_SizeY" ("group name in (Untitled)"), 9:w15) -> (4:w48:refnum<k34>)  [unwired: 3 in, 3 out]
  n68 = call "PECT_GateConverse.vi"("Gate 2"="Gate 2", "Gate 1"="Gate 1", "Freq_Sampling_SizeX_SizeY"=w15) -> ("Length T/2"=w34:i32, "Length"=w35:i32, "Start 2"=w36:i32, "Start 1"=w37:i32)  [unwired: 4 in, 1 out]
  n69 = Obtain Queue(max queue size (-1, unlimited)=10000, name (unnamed)="data DAQ", element data type=dbl[] [] ("data")) -> (queue out=w64:refnum<queue>)  [unwired: 2 in, 2 out]
  n70 = Initialize Array(0.0 ("element"), w44) -> (w65:dbl[])
  n71 = Obtain Queue(name (unnamed)="data Extraction", element data type=0.0) -> (queue out=w62:refnum<queue>)  [unwired: 3 in, 2 out]
  n72 = Obtain Queue(max queue size (-1, unlimited)=2 ("최대 큐 크기(-1,제한없음)"), name (unnamed)="2D data", element data type=dbl[][] [] ("initialized array")) -> (queue out=w12:refnum<queue>)  [unwired: 2 in, 2 out]
  n73 = call "Sigma_SetSpeed.vi"("VISA resource name"=w17, "Travel per Pulse (0.004mm)"="Travel per Pulse (mm)", "Min (1mm) 2"="2 Min", "Max (2mm) 2"="2 Max", "Rate (1mm) 2"="2 Rate", "error in (no error)"=w16, "Axis (1)"="W", "Min (1mm)"="1 Min", "Max (2mm)"="1  Max", "Rate (1mm)"="1 Rate") -> ("VISA resource name out"=w109:refnum<visa-resource-name>, "error out"=w110:errorcluster)  [unwired: 8 in]
  n74 = case shown="\"                          Scan mode                      \", Default" "Tab Control 2" {
    tunnel: w51 -> [w245 w487]
    tunnel: [w244 w486] -> w75
    tunnel: [w243 w485] -> w74
    tunnel: w65 -> [w240 w484]
    tunnel: w9 -> [w242 w483]
    tunnel: w34 -> [w241 w482]
    tunnel: w64 -> [w239 _]
    tunnel: w62 -> [w218 _]
    tunnel: w47 -> [w213 _]
    tunnel: w5 -> [w214 _]
    tunnel: w35 -> [w226 w480]
    tunnel: w37 -> [w225 w479]
    tunnel: w36 -> [w224 w478]
    tunnel: w48 -> [w223 _]
    tunnel: "Waveform" ("group name in (Untitled)") -> [w220 _]
    tunnel: w12 -> [w215 _]
    frame "                          Scan mode                      ", Default {
      # "Column"
      # "Row"
      n75 = Initialize Array(0.0 ("element"), w213, w214) -> (w232:dbl[][])
      n76 = local read "3D Surface"() -> (w227:refnum<k7>)
      n77 = Matrix Size(0:w232) -> (1:w233:i32, 2:w234:i32)
      n78 = Decrement(x=w233) -> (x-1=w237:i32)
      n79 = Decrement(x=w234) -> (x-1=w236:i32)
      n80 = call "Surface_AxesScale.vi"("Y-axis Max"=w236, "X-axis max"=w237, "3D Surface"=w227, "Auto Scale"=FALSE) -> ()  [unwired: 8 in]
      n81 = while {
        shift-right: [w290] -> _
        shift-left: 0 -> [w292]
        shift-right: [w289] -> _
        shift-left: 0 -> [w291]
        tunnel: w218 -> [w288]
        shift-right: [w280] -> w211
        shift-left: w232 -> [w287]
        shift-right: [w283] -> _
        shift-left: TRUE ("Output Direction") -> [w284]
        tunnel: w215 -> [w282]
        tunnel: [w281] -> w216
        stop <- w285 stop-if-true
        n82 = local read "Scan"() -> (w279:bool)
        n83 = local read "Completed"() -> (w278:bool)
        n84 = Compound Arithmetic op=AND(invert w279, invert w278) -> (w277:bool)
        n85 = case shown="True" w277 {
          tunnel: w292 -> [w308 w354]
          tunnel: w291 -> [w307 w353]
          tunnel: [w306 w354] -> w290
          tunnel: [w300 w353] -> w289
          tunnel: w288 -> [w305 w346]
          tunnel: w287 -> [w304 w350]
          tunnel: [w297 w333] -> w280
          tunnel: [w303 _] -> w276
          tunnel: w284 -> [w302 w352]
          tunnel: [w301 w352] -> w283
          tunnel: w282 -> [w298 w335]
          tunnel: [w296 w346] -> w281
          frame False {
            n86 = Dequeue Element(queue=w305) -> (queue out=w296:refnum<queue>, element=w299:dbl)  [unwired: 2 in, 2 out]
            n87 = call "EletoMatr_1channel.vi"("Input Array X"=w304, "Input data"=w299, "In Row"=w308, "In Column"=w307, "Input Direction"=w302) -> ("Completed"=w303:bool, "Out Array X"=w297:dbl[][], "Out Row"=w306:i32, "Output Direction"=w301:bool, "Out Column"=w300:i32)  [unwired: 6 in]
            n88 = Lossy Enqueue Element(queue=w298, element=w297) -> ()  [unwired: 1 in, 4 out]
          }
          frame True {
            n89 = local read "Gate 1"() -> (w349:dbl)
            n90 = local read "Gate 2"() -> (w348:dbl)
            n91 = Wait Until Next ms Multiple(millisecond multiple=u32 100 ("ms 배수")) -> ()  [unwired: 1 out]
            n92 = local read "Offset"() -> (w340:bool)
            n93 = call "TDMS_Open.vi"("Offset"=w340, "Gate 2"=w348, "Gate 1"=w349, "Input 2D"=w350, "Open"="Open tdms") -> ("Output 2D"=w313:dbl[][])  [unwired: 5 in, 1 out]
            n94 = case shown="True" "Open tdms" {
              tunnel: w313 -> [_ w355]
              frame False {
              }
              frame True {
                n95 = global write "Global_data.vi" "global 2d graph"(w355) -> ()
              }
            }
            n96 = call "RepairLine.vi"("Repair Line Col"="Repair Line Col", "Repair Line Row"="Repair Line Row", "Line Col"="Line Col", "Line Row"="Line Row", "Array In"=w313) -> ("Array Repaired"=w327:dbl[][])  [unwired: 6 in]
            n97 = call "CSV Open.vi"("2D Array In"=w327, "Open"="Open csv") -> ("2D Array Out"=w334:dbl[][])  [unwired: 9 in]
            n98 = call "Backdata.vi"("Backindex"="Backindex", "Array in"=w334, "Backdata"="Backdata") -> ("Array out"=w316:dbl[][])
            n99 = call "TrimXY.vi"("X-max"="Y-max", "X-min"="Y-min", "Y-max"="X-max", "Y-min"="X-min", "Array In"=w316, "Trim data"="Trim data") -> ("Array Trim Out"=w315:dbl[][])  [unwired: 5 in]
            n100 = global read "Global_data.vi" "global 2d graph"() -> (w310:dbl[][])
            n101 = call "Inverse.vi"(10:"Inverse"=w315, 11:"Inverse"="Inverse") -> ("Array out"=w311:dbl[][])  [unwired: 9 in]
            n102 = call "Return data.vi"("Array Return"=w310, "Array Input"=w311, "Return"="Return") -> ("Array out"=w309:dbl[][])  [unwired: 8 in]
            n103 = call "Abs.vi"("Input"=w309, "Abs"="Abs") -> ("Array out"=w339:dbl[][])  [unwired: 9 in]
            n104 = call "DiffX.vi"("Array in"=w339, "DiffX"="DiffX") -> ("Array out"=w344:dbl[][])  [unwired: 1 in]
            n105 = call "DiffY.vi"("Array in"=w344, "DiffY"="DiffY") -> ("Array out"=w342:dbl[][])  [unwired: 1 in]
            n106 = call "Odd.vi"("Odd"="Odd", "Array In"=w342) -> ("Array Out"=w331:dbl[][])  [unwired: 9 in]
            n107 = call "Filter_Lowpass - 2D.vi"("Filter"="Filter", "Input 2D"=w331, "low cutoff freq: fl"="low cutoff freq: fl") -> ("Output"=w330:dbl[][])  [unwired: 6 in]
            n108 = case shown="True" TRUE {
              tunnel: w330 -> [w356 w357]
              tunnel: [w356 w357] -> w333
              tunnel: w335 -> [_ w358]
              frame False {
              }
              frame True {
                n109 = local read "3D Surface"() -> (w362:refnum<k7>)
                n110 = Matrix Size(0:w357) -> (1:w363:i32, 2:w360:i32)
                n111 = Decrement(x=w363) -> (x-1=w361:i32)
                n112 = Decrement(x=w360) -> (x-1=w359:i32)
                n113 = call "Surface_AxesScale.vi"("Y-axis Max"=w359, "X-axis max"=w361, "3D Surface"=w362, "Auto Scale"=FALSE) -> ()  [unwired: 8 in]
                n114 = Lossy Enqueue Element(queue=w358, element=w357) -> ()  [unwired: 1 in, 4 out]
              }
            }
          }
        }
        n115 = case shown="True" w276 {
          selector: w276 -> [w293 w294]
          tunnel: [w293 w294] -> w275
          frame False {
          }
          frame True {
            n116 = Wait (ms)(milliseconds to wait=u32 200) -> ()  [unwired: 1 out]
          }
        }
        "Completed" <- w275
        n117 = local read "Stop Scan"() -> (w286:bool)
        n118 = Compound Arithmetic op=OR(w275, w286) -> (w285:bool)
        "No. Y" <- w291
        "No. X" <- w292
      }
      n119 = while {
        tunnel: w245 -> [w373]
        tunnel: [w372] -> w244
        tunnel: [w371] -> w243
        tunnel: w242 -> [w370]
        tunnel: w239 -> [w369]
        stop <- w365 stop-if-true
        n120 = case shown="True" "Scan" {
          tunnel: w373 -> [w375 w380]
          tunnel: [w375 w379] -> w372
          tunnel: [w374 w378] -> w371
          tunnel: w370 -> [w374 w377]
          tunnel: w369 -> [_ w376]
          frame False {
          }
          frame True {
            n121 = while {
              tunnel: w380 -> [w390]
              tunnel: [w393] -> w379
              tunnel: [w392] -> w378
              tunnel: w377 -> [w389]
              tunnel: w376 -> [w391]
              stop <- w381 stop-if-true
              n122 = First Call?() -> (First Call?: T/F=w386:bool)
              n123 = case shown="True" w386 {
                tunnel: w390 -> [w394 w399]
                tunnel: w389 -> [w395 w398]
                tunnel: [w394 w397] -> w388
                tunnel: [w395 w396] -> w387
                frame False {
                }
                frame True {
                  n124 = call <vilib>:"DAQmx Start Task.vi"("task/channels in"=w399, "error in"=w398) -> ("task out"=w397:refnum<k21>, "error out"=w396:errorcluster)  [unwired: 12 in]
                }
              }
              n125 = call-poly <vilib>:"DAQmx Read.vi"("task/channels in"=w388, "error in"=w387) -> ("task out"=w393:refnum<k21>, "data"=w385:dbl[], "error out"=w392:errorcluster)  [unwired: 11 in]
              n126 = Enqueue Element(queue=w391, element=w385) -> ()  [unwired: 2 in, 3 out]
              n127 = Unbundle By Name(w392) -> ("status"=w382:bool)
              n128 = local read "Completed"() -> (w384:bool)
              n129 = local read "Stop Scan"() -> (w383:bool)
              n130 = Compound Arithmetic op=OR(w382, w384, w383) -> (w381:bool)
            }
          }
        }
        n131 = local read "Completed"() -> (w366:bool)
        n132 = local read "Stop Scan"() -> (w367:bool)
        n133 = Compound Arithmetic op=OR(w366, w367) -> (w365:bool)
      }
      n134 = while {
        shift-right: [w416] -> _
        shift-left: w240 -> [w420]
        tunnel: w240 -> [w419]
        tunnel: w241 -> [w418]
        tunnel: w239 -> [w417]
        tunnel: w218 -> [w415]
        shift-right: [w412] -> _
        shift-left: 0 -> [w413]
        tunnel: w226 -> [w411]
        tunnel: w225 -> [w410]
        tunnel: w224 -> [w409]
        tunnel: w223 -> [w408]
        tunnel: [w407] -> w222
        tunnel: [w406] -> w221
        tunnel: w220 -> [w405]
        shift-right: [w403] -> _
        shift-left: 0 -> [w404]
        stop <- w400 stop-if-true
        n135 = local read "Scan"() -> (w414:bool)
        n136 = case shown="True" w414 {
          tunnel: w420 -> [w425 w438]
          tunnel: w419 -> [_ w444]
          tunnel: w418 -> [_ w443]
          tunnel: w417 -> [_ w442]
          tunnel: [w425 w441] -> w416
          tunnel: w415 -> [_ w440]
          tunnel: w413 -> [w424 w436]
          tunnel: [w424 w435] -> w412
          tunnel: w411 -> [_ w434]
          tunnel: w410 -> [_ w433]
          tunnel: w409 -> [_ w432]
          tunnel: w408 -> [w422 w431]
          tunnel: [w422 w430] -> w407
          tunnel: [_ w429] -> w406
          tunnel: w405 -> [_ w428]
          tunnel: w404 -> [w421 w427]
          tunnel: [w421 w426] -> w403
          frame False {
            n137 = Wait Until Next ms Multiple(millisecond multiple=u32 100 ("ms 배수")) -> ()  [unwired: 1 out]
          }
          frame True {
            n138 = local read "Pulser Cycles"() -> (w437:i32)
            n139 = Increment(x=w436) -> (x+1=w435:i32)
            n140 = Dequeue Element(queue=w442) -> (element=w439:dbl[])  [unwired: 2 in, 3 out]
            n141 = Quotient & Remainder(x=w435, y=w437) -> (x-y*floor(x/y)=w445:i32)  [unwired: 1 out]
            n142 = Add(x=w439, y=w438) -> (x+y=w447:dbl[])
            n143 = Equal To 0?(x=w445) -> (x = 0?=w446:bool)
            n144 = case shown="True" w446 {
              tunnel: w437 -> [_ w468]
              tunnel: w447 -> [w450 w466]
              tunnel: [w450 w469] -> w441
              tunnel: w444 -> [_ w469]
              tunnel: w443 -> [_ w462]
              tunnel: w440 -> [_ w467]
              tunnel: w434 -> [_ w463]
              tunnel: w433 -> [_ w465]
              tunnel: w432 -> [_ w464]
              tunnel: w431 -> [w449 w456]
              tunnel: [w449 w453] -> w430
              tunnel: [_ w452] -> w429
              tunnel: w428 -> [_ w455]
              tunnel: w427 -> [w448 w458]
              tunnel: [w448 w457] -> w426
              frame False {
                n145 = disable-structure shown="비활성화" {
                  frame Disabled {
                    n146 = Wait Until Next ms Multiple(millisecond multiple=u32 100 ("ms 배수")) -> ()  [unwired: 1 out]
                  }
                  frame Enabled {
                  }
                }
              }
              frame True {
                n147 = Divide(x=w466, y=w468) -> (x/y=w454:dbl[])
                n148 = local read "Offset"() -> (w461:bool)
                n149 = local read "Motor Pulse Count"() -> (w457:i32)
                n150 = call "PECT_Feature extraction.vi"("Length T/2"=w462, "Offset"=w461, "Length"=w463, "Start 2"=w464, "Start 1"=w465, "Pulse signal in"=w454) -> ("Feature extraction out"=w460:dbl)  [unwired: 5 in]
                n151 = Not Equal?(x=w457, y=w458) -> (x != y?=w459:bool)
                n152 = case shown="True" w459 {
                  tunnel: w467 -> [_ w477]
                  tunnel: w460 -> [_ w476]
                  tunnel: w456 -> [w470 w475]
                  tunnel: w455 -> [_ w474]
                  tunnel: w454 -> [_ w473]
                  tunnel: [w470 w472] -> w453
                  tunnel: [_ w471] -> w452
                  frame False {
                  }
                  frame True {
                    n153 = TDMS Write(0:w475, 5:w474, 9:w473) -> (4:w472:refnum<k34>, 15:w471:errorcluster)  [unwired: 3 in, 2 out]
                    n154 = Enqueue Element(queue=w477, element=w476) -> ()  [unwired: 2 in, 3 out]
                  }
                }
              }
            }
          }
        }
        n155 = local read "Completed"() -> (w402:bool)
        n156 = local read "Stop Scan"() -> (w401:bool)
        n157 = Compound Arithmetic op=OR(w402, w401) -> (w400:bool)
        "No.data" <- w413
      }
      n158 = while {
        tunnel: w215 -> [w272]
        tunnel: w214 -> [_]
        tunnel: w213 -> [_]
        tunnel: [w269] -> w212
        stop <- w270 stop-if-true
        n159 = local read "No. Y"() -> (w266:i32)
        n160 = call "CursorPosition.vi"("Cursor No."=1.0, "Cursor"="Cursor", "3D Surface Analysis"="3D Surface") -> ("Cursor Y"=w261:dbl)  [unwired: 6 in, 2 out]
        n161 = Dequeue Element(queue=w272) -> (queue out=w269:refnum<queue>, element=w268:dbl[][])  [unwired: 2 in, 2 out]
        n162 = Add(x=w266, y=w261) -> (x+y=w265:dbl)
        n163 = Index Array(array=w268, index (col)=w265) -> (element=→"Feature extraction scan":dbl[])  [unwired: 1 in]
        n164 = call <vilib>:"3D Surface.vi"("z matrix"=w268, "3D graph"="3D Surface") -> ()  [unwired: 8 in, 2 out]
        n165 = local read "Completed"() -> (w267:bool)
        n166 = local read "Stop Scan"() -> (w271:bool)
        n167 = Compound Arithmetic op=OR(w267, w271) -> (w270:bool)
        n168 = Wait Until Next ms Multiple(millisecond multiple=u32 100 ("ms 배수")) -> ()  [unwired: 1 out]
      }
      n169 = Release Queue(queue=w212) -> ()  [unwired: 2 in, 3 out]
      n170 = while {
        stop <- w250 stop-if-true
        n171 = event shown="[2] \"Max\", \"Min\", \"ColorMapAutoScale\": Value Change" {
          selector: _ -> [_ _ _]
          dyn-events: _ -> [_ _ _]
          timeout: _ -> [_ _ _]
          tunnel: [_ w254 _] -> w250
          event "Plot style", "ViewMode": Value Change {
            n172 = event-data() -> ()  [unwired: 1 in, 2 out]
            n173 = local read "3D Surface"() -> (w253:refnum<k7>)
            n174 = property class="CWGraph3D"(reference=w253, "ViewMode"="ViewMode") -> ()  [unwired: 1 in, 2 out]
            n175 = call <vilib>:"Basic Properties.vi"("3D graph"=w253, "plot style"="Plot style") -> ()  [unwired: 12 in, 2 out]
          }
          event "Stop Scan": Value Change {
            n176 = event-data() -> ()  [unwired: 1 in, 5 out]
            n177 = local read "Stop Scan"() -> (w254:bool)
          }
          event "Max", "Min", "ColorMapAutoScale": Value Change {
            n178 = event-data() -> ()  [unwired: 1 in, 5 out]
            n179 = local read "3D Surface"() -> (w255:refnum<k7>)
            n180 = call "Surface_ColorScale.vi"("ColorMapAutoScale"="ColorMapAutoScale", "Min"="Min", "Max"="Max", "3D Surface_"=w255) -> ("Min 2"=w259:dbl, "Max 2"=w258:dbl)  [unwired: 1 in, 2 out]
            n181 = local write "Max"(w258) -> ()
            n182 = local write "Min"(w259) -> ()
          }
        }
      }
      n183 = TDMS Close(8:w221, 11:w222) -> (0:w219:errorcluster)  [unwired: 1 out]
      n184 = call <vilib>:"Simple Error Handler.vi"("error in (no error)"=w219) -> ()  [unwired: 2 in, 7 out]
      n185 = Release Queue(queue=w216) -> ()  [unwired: 2 in, 3 out]
      n186 = while {
        tunnel: w211 -> [w248]
        stop <- w247 stop-if-true
        n187 = call "CSV Save.vi"("Array"=w248, "Save Button"="Save Scan mode") -> ()  [unwired: 9 in, 1 out]
        n188 = Wait Until Next ms Multiple(millisecond multiple=u32 100 ("ms 배수")) -> ()  [unwired: 1 out]
        n189 = local read "Stop Scan"() -> (w247:bool)
      }
    }
    frame "                    Test mode                   " {
      n190 = while {
        tunnel: w487 -> [w497]
        tunnel: w483 -> [w496]
        tunnel: [w515] -> w485
        tunnel: [w516] -> w486
        shift-right: [w511] -> _
        shift-left: w484 -> [w512]
        tunnel: w484 -> [w510]
        shift-right: [w508] -> _
        shift-left: _ -> [w507]
        tunnel: w482 -> [w506]
        shift-right: [w505] -> _
        shift-left: _ -> [w504]
        shift-right: [w501] -> _
        shift-left: 1 ("Average") -> [w500]
        tunnel: w480 -> [w493]
        tunnel: w479 -> [w492]
        tunnel: w478 -> [w491]
        stop <- w517 stop-if-true
        n191 = First Call?() -> (First Call?: T/F=w498:bool)
        n192 = case shown="True" w498 {
          tunnel: w497 -> [w518 w523]
          tunnel: w496 -> [w519 w522]
          tunnel: [w518 w521] -> w495
          tunnel: [w519 w520] -> w494
          frame False {
          }
          frame True {
            n193 = call <vilib>:"DAQmx Start Task.vi"("task/channels in"=w523, "error in"=w522) -> ("task out"=w521:refnum<k21>, "error out"=w520:errorcluster)  [unwired: 12 in]
          }
        }
        n194 = local read "Pulser Cycles"() -> (w499:i32)
        n195 = call-poly <vilib>:"DAQmx Read.vi"("task/channels in"=w495, "timeout"=-1.0, "error in"=w494) -> ("task out"=w516:refnum<k21>, "data"=w489:waveform(dbl), "error out"=w515:errorcluster)  [unwired: 10 in]
        n196 = Unbundle By Name(w489) -> ("Y"=w488:dbl[])
        n197 = Quotient & Remainder(x=w500, y=w499) -> (x-y*floor(x/y)=w513:i32)  [unwired: 1 out]
        n198 = Equal To 0?(x=w513) -> (x = 0?=w490:bool)
        n199 = Add(x=w488, y=w512) -> (x+y=w509:dbl[])
        n200 = case shown="True" w490 {
          tunnel: w499 -> [_ w543]
          tunnel: w489 -> [_ w536]
          tunnel: w509 -> [w528 w549]
          tunnel: [w528 w548] -> w511
          tunnel: w510 -> [_ w548]
          tunnel: [w527 w546] -> w508
          tunnel: w507 -> [w527 w547]
          tunnel: w506 -> [_ w530]
          tunnel: [w526 w544] -> w505
          tunnel: w504 -> [w526 w545]
          tunnel: [w524 1 ("Average")] -> w501
          tunnel: w500 -> [w525 _]
          tunnel: w493 -> [_ w531]
          tunnel: w492 -> [_ w533]
          tunnel: w491 -> [_ w532]
          frame False {
            n201 = Increment(x=w525) -> (x+1=w524:i32)
          }
          frame True {
            n202 = Divide(x=w549, y=w543) -> (x/y=w529:dbl[])
            n203 = Bundle By Name(cluster=w536, "Y"=w529) -> (w537:waveform(dbl))
            n204 = xnode "Spectral Measurements"("신호"=w537) -> ("PSD"=w539:cluster{"f0":dbl, "df":dbl, "magnitude":dbl[]})  [unwired: 1 in, 1 out]
            n205 = call "PECT_Feature extraction.vi"("Length T/2"=w530, "Offset"="Offset", "Length"=w531, "Start 2"=w532, "Start 1"=w533, "Pulse signal in"=w529) -> ("Feature extraction out"=→"Feature Extraction":dbl)  [unwired: 5 in]
            n206 = case shown="True" "2 Plots" {
              tunnel: [w553 w559] -> w541
              tunnel: w547 -> [_ w558]
              tunnel: [w552 w558] -> w546
              tunnel: w537 -> [w552 w554]
              tunnel: w539 -> [w550 w556]
              tunnel: [w551 w557] -> w538
              tunnel: w545 -> [_ w555]
              tunnel: [w550 w555] -> w544
              frame False {
                n207 = Build Array(w550, w550) -> (w551:cluster{"f0":dbl, "df":dbl, "magnitude":dbl[]}[])
                n208 = Build Array(w552, w552) -> (w553:waveform(dbl)[])
              }
              frame True {
                n209 = Build Array(w555, w556) -> (w557:cluster{"f0":dbl, "df":dbl, "magnitude":dbl[]}[])
                n210 = Build Array(w558, w554) -> (w559:waveform(dbl)[])
              }
            }
            "Power spectral density" <- w538
            "Hall sensors signal" <- w541
          }
        }
        n211 = local read "Stop Scan"() -> (w503:bool)
        n212 = Unbundle By Name(w515) -> ("status"=w514:bool)
        n213 = Or(x=w514, y=w503) -> (x .or. y?=w517:bool)
      }
    }
  }
  n214 = call <vilib>:"DAQmx Start Task.vi"("task/channels in"=w20, "error in"=w21) -> ("task out"=w22:refnum<k21>, "error out"=w8:errorcluster)  [unwired: 12 in]
  n215 = while {
    tunnel: w22 -> [w579]
    tunnel: w8 -> [w578]
    tunnel: [w570] -> w29
    tunnel: [w577] -> w28
    tunnel: [w569] -> _
    tunnel: w6 -> [w569]
    stop <- w571 stop-if-true
    n216 = call-poly <vilib>:"DAQmx Read.vi"("task/channels in"=w579, "error in"=w578) -> ("task out"=w577:refnum<k21>, "data"=→"Motor Pulse Count":u32, "error out"=w570:errorcluster)  [unwired: 11 in]
    n217 = Wait Until Next ms Multiple(millisecond multiple=u32 10 ("milliseconds to wait")) -> ()  [unwired: 1 out]
    n218 = local read "Completed"() -> (w572:bool)
    n219 = Unbundle By Name(w570) -> ("status"=w574:bool)
    n220 = local read "Stop Scan"() -> (w573:bool)
    n221 = Compound Arithmetic op=OR(w574, w572, w573) -> (w571:bool)
  }
  n222 = while {
    shift-right: [w595] -> _
    shift-left: T4."No Scan" -> [w596]
    shift-right: [w591] -> _
    shift-left: 0.0 ("Current  Position (mm)") -> [w590]
    shift-right: [w589] -> _
    shift-left: 0.0 ("Current  Position (mm)") -> [w588]
    shift-right: [w587] -> _
    shift-left: 0.0 ("Current  Position (mm)") -> [w586]
    shift-right: [w585] -> _
    shift-left: 0.0 ("Current  Position (mm)") -> [w584]
    shift-right: [w592] -> w41
    shift-left: w109 -> [w594]
    shift-right: [w582] -> w42
    shift-left: w110 -> [w593]
    tunnel: w6 -> [_]
    stop <- w580 stop-if-true
    n223 = case shown="\"Wait to destinatioin Y\"" w596 {
      selector: w596 -> [w607 _ _ _ _]
      tunnel: [w608 T4."Wait to destination X" w672 w706 w745] -> w595
      tunnel: w594 -> [w602 w641 w666 w708 w736]
      tunnel: w593 -> [w601 w640 w665 w707 w735]
      tunnel: [w604 w643 w671 w702 w742] -> w592
      tunnel: [w603 w642 w670 w701 w741] -> w582
      tunnel: [w600 w648 w669 w705 w748] -> w591
      tunnel: w590 -> [w598 w648 w657 w705 w748]
      tunnel: [w606 w647 w674 w704 w747] -> w589
      tunnel: w588 -> [w597 w647 w674 w704 w747]
      tunnel: [w599 w646 w667 w690 w744] -> w587
      tunnel: w586 -> [_ w646 w667 w690 w730]
      tunnel: [w605 w645 w675 w703 w743] -> w585
      tunnel: w584 -> [_ w645 w675 w703 w743]
      frame "No Scan", Default {
        n224 = local read "Scan"() -> (w609:bool)
        n225 = case shown="True" w609 {
          tunnel: [w615 T4."Move X"] -> w608
          tunnel: w607 -> [w615 _]
          tunnel: w602 -> [w614 w621]
          tunnel: w601 -> [w613 w620]
          tunnel: [w614 w626] -> w604
          tunnel: [w613 w625] -> w603
          tunnel: [w612 w617] -> w600
          tunnel: [w611 w616] -> w599
          tunnel: w598 -> [w612 _]
          tunnel: w597 -> [w611 _]
          frame False {
            n226 = Wait (ms)(milliseconds to wait=u32 100) -> ()  [unwired: 1 out]
          }
          frame True {
            n227 = local read "Cur. Pos X"() -> (w623:dbl)
            n228 = local read "Cur. Pos Y"() -> (w624:dbl)
            n229 = local read "Travel per Pulse (mm)"() -> (w622:dbl)
            n230 = call "Sigma_GetPos.vi"("VISA resource name"=w621, "Travel per Pulse (mm)"=w622, "Init Pos X (mm)"=w623, "Init  Pos Y (mm)"=w624, "error in (no error)"=w620) -> ("Pos X (mm)"=w617:dbl, "Pos Y (mm)"=w616:dbl, "VISA resource name out"=w619:refnum<visa-resource-name>, "error out"=w618:errorcluster)  [unwired: 6 in, 1 out]
            "Start Pos. X" <- w617
            "Start. Pos.Y" <- w616
            n231 = local write "Cur. Pos X"(w617) -> ()
            n232 = local write "Cur. Pos Y"(w616) -> ()
            n233 = local read "Step X"() -> (w630:dbl)
            n234 = local read "Travel per Pulse (mm)"() -> (w629:dbl)
            n235 = local write "Direction (+)"(TRUE ("Direction (+)")) -> ()
            n236 = local write "Move X"(TRUE ("Move X")) -> ()
            n237 = call "Sigma_TriggerOut.vi"("Axis(1)"=1, "error in (no error)"=w618, "Trigger distance (mm)"=w630, "Travel per Pulse (mm)"=w629, "VISA resource name"=w619) -> ("error out"=w627:errorcluster, "VISA resource name out"=w628:refnum<visa-resource-name>)  [unwired: 5 in]
            n238 = flat-sequence {
              tunnel: [w637] -> w626
              tunnel: w628 -> [w637]
              tunnel: [w636] -> w625
              tunnel: w627 -> [w636]
              frame #0 {
                n239 = Wait (ms)(milliseconds to wait=u32 100) -> ()  [unwired: 1 out]
              }
            }
          }
        }
        n240 = local read "X-length"() -> (w606:dbl)
        n241 = local read "Step Y"() -> (w605:dbl)
      }
      frame "Move X" {
        n242 = local read "Travel per Pulse (mm)"() -> (w650:dbl)
        n243 = local read "X-length"() -> (w651:dbl)
        n244 = call "Sigma_MoveAbs.vi"("Direction (+)"="Direction (+)", "Axis (1)"=1, "error in (no error)"=w640, "Travel (1mm)"=w651, "Travel per Pulse (0.004mm)"=w650, "VISA resource name"=w641) -> ("error out"=w638:errorcluster, "VISA resource name out"=w639:refnum<visa-resource-name>)  [unwired: 4 in]
        n245 = flat-sequence {
          tunnel: [w655] -> w643
          tunnel: w639 -> [w655]
          tunnel: [w654] -> w642
          tunnel: w638 -> [w654]
          frame #0 {
            n246 = Wait (ms)(milliseconds to wait=u32 100) -> ()  [unwired: 1 out]
          }
        }
      }
      frame "Wait to destination X" {
        n247 = local read "Cur. Pos X"() -> (w662:dbl)
        n248 = local read "Cur. Pos Y"() -> (w661:dbl)
        n249 = local read "Travel per Pulse (mm)"() -> (w668:dbl)
        n250 = call "Sigma_GetPos.vi"("VISA resource name"=w666, "Travel per Pulse (mm)"=w668, "Init Pos X (mm)"=w662, "Init  Pos Y (mm)"=w661, "error in (no error)"=w665) -> ("Pos X (mm)"=w656:dbl, "Pos Y (mm)"=w660:dbl, "VISA resource name out"=w664:refnum<visa-resource-name>, "error out"=w663:errorcluster)  [unwired: 6 in, 1 out]
        n251 = Absolute Value(x=w674) -> (abs(x)=w676:dbl)
        n252 = local write "Cur. Pos X"(w656) -> ()
        n253 = local write "Cur. Pos Y"(w660) -> ()
        n254 = Subtract(x=w656, y=w657) -> (x-y=w678:dbl)
        n255 = Absolute Value(x=w678) -> (abs(x)=w677:dbl)
        n256 = Subtract(x=w677, y=w676) -> (x-y=w659:dbl)
        n257 = call "Convert Double Precision.vi"("Input"=w659) -> ("Output"=w658:dbl)  [unwired: 10 in]
        n258 = Greater Or Equal To 0?(x=w658) -> (x >= 0?=w673:bool)
        n259 = case shown="True" w673 {
          tunnel: [T4."Wait to destination X" T4."Move Y"] -> w672
          tunnel: w664 -> [w681 w685]
          tunnel: w663 -> [w680 w684]
          tunnel: [w681 w685] -> w671
          tunnel: [w680 w684] -> w670
          tunnel: [w679 w686] -> w669
          tunnel: w657 -> [w679 _]
          frame False {
            n260 = disable-structure shown="비활성화" {
              frame Disabled {
                n261 = Wait (ms)(milliseconds to wait=u32 100) -> ()  [unwired: 1 out]
              }
              frame Enabled {
              }
            }
          }
          frame True {
            n262 = local read "Cur. Pos X"() -> (w686:dbl)
            n263 = local write "Move X"(FALSE ("Move X")) -> ()
          }
        }
      }
      frame "Move Y" {
        n264 = local read "Y-length"() -> (w693:dbl)
        n265 = local read "Step Y"() -> (w691:dbl)
        n266 = local read "Start. Pos.Y"() -> (w696:dbl)
        n267 = Subtract(x=w693, y=w691) -> (x-y=w692:dbl)
        n268 = Subtract(x=w696, y=w690) -> (x-y=w700:dbl)
        n269 = Absolute Value(x=w692) -> (abs(x)=w698:dbl)
        n270 = Absolute Value(x=w700) -> (abs(x)=w699:dbl)
        n271 = Subtract(x=w699, y=w698) -> (x-y=w694:dbl)
        n272 = local write "Move X"(FALSE ("Move X")) -> ()
        n273 = call "Convert Double Precision.vi"("Input"=w694) -> ("Output"=w695:dbl)  [unwired: 10 in]
        n274 = Greater Or Equal To 0?(x=w695) -> (x >= 0?=w689:bool)
        n275 = case shown="True" w689 {
          tunnel: w708 -> [w717 w727]
          tunnel: w707 -> [w716 w725]
          tunnel: [T4."Wait to destinatioin Y" T4."No Scan"] -> w706
          tunnel: [w711 w726] -> w702
          tunnel: [w710 w724] -> w701
          frame False {
            n276 = local read "Travel per Pulse (mm)"() -> (w715:dbl)
            n277 = local read "Step Y"() -> (w718:dbl)
            n278 = call "Sigma_MoveAbs.vi"("Direction (+)"=TRUE, "Axis (1)"=2, "error in (no error)"=w716, "Travel (1mm)"=w718, "Travel per Pulse (0.004mm)"=w715, "VISA resource name"=w717) -> ("error out"=w712:errorcluster, "VISA resource name out"=w713:refnum<visa-resource-name>)  [unwired: 4 in]
            n279 = flat-sequence {
              tunnel: [w722] -> w711
              tunnel: w713 -> [w722]
              tunnel: [w721] -> w710
              tunnel: w712 -> [w721]
              frame #0 {
                n280 = Wait (ms)(milliseconds to wait=u32 100) -> ()  [unwired: 1 out]
              }
            }
          }
          frame True {
            n281 = call "Sigma_TriggerOff.vi"("error in (no error)"=w725, "VISA resource name"=w727) -> ("error out"=w724:errorcluster, "VISA resource name out"=w726:refnum<visa-resource-name>)  [unwired: 8 in]
            n282 = local write "Scan"(FALSE ("Move X")) -> ()
          }
        }
      }
      frame "Wait to destinatioin Y" {
        n283 = local read "Cur. Pos X"() -> (w739:dbl)
        n284 = local read "Cur. Pos Y"() -> (w738:dbl)
        n285 = local read "Travel per Pulse (mm)"() -> (w740:dbl)
        n286 = call "Sigma_GetPos.vi"("VISA resource name"=w736, "Travel per Pulse (mm)"=w740, "Init Pos X (mm)"=w739, "Init  Pos Y (mm)"=w738, "error in (no error)"=w735) -> ("Pos X (mm)"=w737:dbl, "Pos Y (mm)"=w729:dbl, "VISA resource name out"=w734:refnum<visa-resource-name>, "error out"=w733:errorcluster)  [unwired: 6 in, 1 out]
        n287 = Absolute Value(x=w743) -> (abs(x)=w749:dbl)
        n288 = Subtract(x=w729, y=w730) -> (x-y=w751:dbl)
        n289 = local write "Cur. Pos X"(w737) -> ()
        n290 = local write "Cur. Pos Y"(w729) -> ()
        n291 = Absolute Value(x=w751) -> (abs(x)=w750:dbl)
        n292 = Subtract(x=w750, y=w749) -> (x-y=w732:dbl)
        n293 = call "Convert Double Precision.vi"("Input"=w732) -> ("Output"=w731:dbl)  [unwired: 10 in]
        n294 = Greater Or Equal To 0?(x=w731) -> (x >= 0?=w746:bool)
        n295 = case shown="True" w746 {
          tunnel: [T4."Wait to destinatioin Y" T4."Move X"] -> w745
          tunnel: w730 -> [w754 _]
          tunnel: [w754 w761] -> w744
          tunnel: [w753 w760] -> w742
          tunnel: [w752 w759] -> w741
          tunnel: w734 -> [w753 w760]
          tunnel: w733 -> [w752 w759]
          frame False {
            n296 = disable-structure shown="비활성화" {
              frame Disabled {
                n297 = Wait (ms)(milliseconds to wait=u32 100) -> ()  [unwired: 1 out]
              }
              frame Enabled {
              }
            }
          }
          frame True {
            n298 = local read "Direction (+)"() -> (w758:bool)
            n299 = local read "Cur. Pos Y"() -> (w761:dbl)
            n300 = Not(x=w758) -> (.not. x?=w757:bool)
            n301 = local write "Direction (+)"(w757) -> ()
            n302 = local write "Move X"(TRUE ("Move X")) -> ()
          }
        }
      }
    }
    n303 = Unbundle By Name(w582) -> ("status"=w581:bool)
    n304 = local read "Stop Scan"() -> (w583:bool)
    n305 = Compound Arithmetic op=OR(w581, w583) -> (w580:bool)
  }
  n306 = while {
    shift-right: [w766] -> _
    shift-left: w109 -> [w771]
    shift-right: [w768] -> _
    shift-left: w110 -> [w770]
    stop <- w767 stop-if-true
    n307 = event shown="[0] Timeout" {
      selector: _ -> [_ _ _ _ _ _ _ _ _ _ _]
      dyn-events: _ -> [_ _ _ _ _ _ _ _ _ _ _]
      timeout: 100 -> [_ _ _ _ _ _ _ _ _ _ _]
      tunnel: w771 -> [w776 w809 w822 w825 w840 w855 w870 w887 w899 w909 w921]
      tunnel: w770 -> [w775 w808 w819 w824 w839 w854 w869 w886 w898 w908 w920]
      tunnel: [w774 w809 w821 w827 w842 w857 w872 w884 w897 w911 w923] -> w766
      tunnel: [w773 w808 w820 w826 w841 w856 w871 w883 w896 w910 w922] -> w768
      tunnel: [_ "Stop Scan" _ _ _ _ _ _ _ _ _] -> w765
      event Timeout {
        n308 = event-data() -> ()  [unwired: 1 in, 2 out]
        n309 = local read "Scan"() -> (w772:bool)
        n310 = case shown="False" w772 {
          tunnel: w776 -> [w788 w807]
          tunnel: w775 -> [w787 w806]
          tunnel: [w786 w807] -> w774
          tunnel: [w785 w806] -> w773
          frame False {
            # "Stop at LS"
            n311 = local read "Cur. Pos X"() -> (w778:dbl)
            n312 = local read "Cur. Pos Y"() -> (w777:dbl)
            n313 = local read "Travel per Pulse (mm)"() -> (w780:dbl)
            n314 = call "Sigma_GetPos.vi"("VISA resource name"=w788, "Travel per Pulse (mm)"=w780, "Init Pos X (mm)"=w778, "Init  Pos Y (mm)"=w777, "error in (no error)"=w787) -> ("Pos X (mm)"=w783:dbl, "Pos Y (mm)"=w784:dbl, "VISA resource name out"=w781:refnum<visa-resource-name>, "State String"=w779:string, "error out"=w782:errorcluster)  [unwired: 6 in]
            n315 = local write "Cur. Pos X"(w783) -> ()
            n316 = local write "Cur. Pos Y"(w784) -> ()
            n317 = case shown="\"W\"" w779 {
              tunnel: [w790 w795 w800 w805] -> w786
              tunnel: [w789 w794 w799 w804] -> w785
              tunnel: w781 -> [w790 w792 w797 w802]
              tunnel: w782 -> [w789 w791 w796 w801]
              frame "K", Default {
              }
              frame "L" {
                n318 = call "Sigma_Stop.vi"("Axis (1)"="1", "error in (no error)"=w791, "VISA resource name"=w792) -> ("error out"=w794:errorcluster, "VISA resource name out"=w795:refnum<visa-resource-name>)  [unwired: 7 in]
              }
              frame "M" {
                n319 = call "Sigma_Stop.vi"("Axis (1)"="2", "error in (no error)"=w796, "VISA resource name"=w797) -> ("error out"=w799:errorcluster, "VISA resource name out"=w800:refnum<visa-resource-name>)  [unwired: 7 in]
              }
              frame "W" {
                n320 = call "Sigma_Stop.vi"("Axis (1)"="W", "error in (no error)"=w801, "VISA resource name"=w802) -> ("error out"=w804:errorcluster, "VISA resource name out"=w805:refnum<visa-resource-name>)  [unwired: 7 in]
              }
            }
          }
          frame True {
          }
        }
      }
      event "Stop Scan": Value Change {
        n321 = event-data() -> ()  [unwired: 1 in, 2 out]
      }
      event "Save Speed": Value Change {
        n322 = event-data() -> ()  [unwired: 1 in, 5 out]
        n323 = local read "Travel per Pulse (mm)"() -> (w811:dbl)
        n324 = local read "1  Max"() -> (w816:dbl)
        n325 = local read "1 Rate"() -> (w815:dbl)
        n326 = local read "2 Rate"() -> (w812:dbl)
        n327 = local read "2 Max"() -> (w813:dbl)
        n328 = local read "1 Min"() -> (w817:dbl)
        n329 = local read "2 Min"() -> (w814:dbl)
        n330 = call "Sigma_SetSpeed.vi"("VISA resource name"=w822, "Travel per Pulse (0.004mm)"=w811, "Min (1mm) 2"=w814, "Max (2mm) 2"=w813, "Rate (1mm) 2"=w812, "error in (no error)"=w819, "Axis (1)"="W", "Min (1mm)"=w817, "Max (2mm)"=w816, "Rate (1mm)"=w815) -> ("VISA resource name out"=w821:refnum<visa-resource-name>, "error out"=w820:errorcluster)  [unwired: 8 in]
      }
      event "Right": Value Change {
        n331 = event-data() -> ()  [unwired: 1 in, 1 out]
        n332 = case shown="True" "Right" {
          tunnel: [w829 w835] -> w827
          tunnel: [w828 w834] -> w826
          tunnel: w825 -> [w829 w837]
          tunnel: w824 -> [w828 w836]
          frame False {
          }
          frame True {
            n333 = local read "Travel per Pulse (mm)"() -> (w831:dbl)
            n334 = local read "Move Distance"() -> (w830:dbl)
            n335 = call "Sigma_MoveAbs.vi"("Direction (+)"=FALSE, "Axis (1)"=1, "error in (no error)"=w836, "Travel (1mm)"=w830, "Travel per Pulse (0.004mm)"=w831, "VISA resource name"=w837) -> ("error out"=w834:errorcluster, "VISA resource name out"=w835:refnum<visa-resource-name>)  [unwired: 4 in]
          }
        }
      }
      event "Left": Value Change {
        n336 = event-data() -> ()  [unwired: 1 in, 1 out]
        n337 = case shown="True" "Left" {
          tunnel: [w844 w851] -> w842
          tunnel: [w843 w850] -> w841
          tunnel: w840 -> [w844 w852]
          tunnel: w839 -> [w843 w849]
          frame False {
          }
          frame True {
            n338 = local read "Travel per Pulse (mm)"() -> (w846:dbl)
            n339 = local read "Move Distance"() -> (w845:dbl)
            n340 = call "Sigma_MoveAbs.vi"("Direction (+)"=TRUE, "Axis (1)"=1, "error in (no error)"=w849, "Travel (1mm)"=w845, "Travel per Pulse (0.004mm)"=w846, "VISA resource name"=w852) -> ("error out"=w850:errorcluster, "VISA resource name out"=w851:refnum<visa-resource-name>)  [unwired: 4 in]
          }
        }
      }
      event "Front": Value Change {
        n341 = event-data() -> ()  [unwired: 1 in, 1 out]
        n342 = case shown="True" "Front" {
          tunnel: [w859 w865] -> w857
          tunnel: [w858 w864] -> w856
          tunnel: w855 -> [w859 w867]
          tunnel: w854 -> [w858 w866]
          frame False {
          }
          frame True {
            n343 = local read "Travel per Pulse (mm)"() -> (w861:dbl)
            n344 = local read "Move Distance"() -> (w860:dbl)
            n345 = call "Sigma_MoveAbs.vi"("Direction (+)"=FALSE, "Axis (1)"=2, "error in (no error)"=w866, "Travel (1mm)"=w860, "Travel per Pulse (0.004mm)"=w861, "VISA resource name"=w867) -> ("error out"=w864:errorcluster, "VISA resource name out"=w865:refnum<visa-resource-name>)  [unwired: 4 in]
          }
        }
      }
      event "Back": Value Change {
        n346 = event-data() -> ()  [unwired: 1 in, 1 out]
        n347 = case shown="True" "Back" {
          tunnel: [w874 w880] -> w872
          tunnel: [w873 w879] -> w871
          tunnel: w870 -> [w874 w882]
          tunnel: w869 -> [w873 w881]
          frame False {
          }
          frame True {
            n348 = local read "Travel per Pulse (mm)"() -> (w876:dbl)
            n349 = local read "Move Distance"() -> (w875:dbl)
            n350 = call "Sigma_MoveAbs.vi"("Direction (+)"=TRUE, "Axis (1)"=2, "error in (no error)"=w881, "Travel (1mm)"=w875, "Travel per Pulse (0.004mm)"=w876, "VISA resource name"=w882) -> ("error out"=w879:errorcluster, "VISA resource name out"=w880:refnum<visa-resource-name>)  [unwired: 4 in]
          }
        }
      }
      event "Home X": Value Change {
        n351 = event-data() -> ()  [unwired: 1 in, 1 out]
        n352 = case shown="True" "Home X" {
          tunnel: [w889 w892] -> w884
          tunnel: [w888 w891] -> w883
          tunnel: w887 -> [w889 w894]
          tunnel: w886 -> [w888 w893]
          frame False {
          }
          frame True {
            n353 = call "Sigma_Home.vi"("Axis (1)"="1", "error in (no error)"=w893, "VISA resource name"=w894) -> ("error out"=w891:errorcluster, "VISA resource name out"=w892:refnum<visa-resource-name>)  [unwired: 7 in]
          }
        }
      }
      event "Home Y": Value Change {
        n354 = event-data() -> ()  [unwired: 1 in, 1 out]
        n355 = case shown="True" "Home Y" {
          tunnel: [w901 w904] -> w897
          tunnel: [w900 w903] -> w896
          tunnel: w899 -> [w901 w906]
          tunnel: w898 -> [w900 w905]
          frame False {
          }
          frame True {
            n356 = call "Sigma_Home.vi"("Axis (1)"="2", "error in (no error)"=w905, "VISA resource name"=w906) -> ("error out"=w903:errorcluster, "VISA resource name out"=w904:refnum<visa-resource-name>)  [unwired: 7 in]
          }
        }
      }
      event "Stop 3": Value Change {
        n357 = event-data() -> ()  [unwired: 1 in, 1 out]
        n358 = case shown="True" "Stop 3" {
          tunnel: [w913 w914] -> w911
          tunnel: [w912 w915] -> w910
          tunnel: w909 -> [w913 w917]
          tunnel: w908 -> [w912 w916]
          frame False {
          }
          frame True {
            n359 = call "Sigma_Stop.vi"("Axis (1)"="W", "error in (no error)"=w916, "VISA resource name"=w917) -> ("error out"=w915:errorcluster, "VISA resource name out"=w914:refnum<visa-resource-name>)  [unwired: 7 in]
          }
        }
      }
      event "Emergency Stop": Value Change {
        n360 = event-data() -> ()  [unwired: 1 in, 1 out]
        n361 = case shown="True" "Emergency Stop" {
          tunnel: [w925 w928] -> w923
          tunnel: [w924 w927] -> w922
          tunnel: w921 -> [w925 w930]
          tunnel: w920 -> [w924 w929]
          frame False {
          }
          frame True {
            n362 = call "Sigma_Stop.vi"("Axis (1)"="E", "error in (no error)"=w929, "VISA resource name"=w930) -> ("error out"=w927:errorcluster, "VISA resource name out"=w928:refnum<visa-resource-name>)  [unwired: 7 in]
          }
        }
      }
    }
    n363 = Unbundle By Name(w768) -> ("status"=w769:bool)
    n364 = Compound Arithmetic op=OR(w769, w765) -> (w767:bool)
  }
  n365 = call <vilib>:"DAQmx Stop Task.vi"("task/channels in"=w28, "error in"=w29) -> ("task out"=w31:refnum<k21>, "error out"=w30:errorcluster)  [unwired: 12 in]
  n366 = call <vilib>:"DAQmx Clear Task.vi"("task in"=w31, "error in"=w30) -> ("error out"=w23:errorcluster)  [unwired: 13 in]
  n367 = call <vilib>:"Simple Error Handler.vi"("error in (no error)"=w23) -> ()  [unwired: 4 in, 5 out]
  n368 = VISA Close(VISA resource name=w41, error in (no error)=w42) -> (error out=w40:errorcluster)
  n369 = call <vilib>:"Simple Error Handler.vi"("error in (no error)"=w40) -> ()  [unwired: 4 in, 5 out]
  n370 = call <vilib>:"DAQmx Clear Task.vi"("task in"=w75, "error in"=w74) -> ("error out"=w81:errorcluster)  [unwired: 13 in]
  n371 = call <vilib>:"Simple Error Handler.vi"("error in (no error)"=w81) -> ()  [unwired: 4 in, 5 out]
  n372 = call <vilib>:"Simple Error Handler.vi"() -> ()  [unwired: 5 in, 5 out]
  "Move X" <- FALSE ("Move X")
